vi "report.vi"() -> ()   [LabVIEW 2019, in "database.lvlib"]
uses:
  database.lvlib
  <vilib>/Utility/NIReport.llb/Report Type.ctl
  <vilib>/addons/_office/_exclsub.llb/font.ctl
  <vilib>/Utility/miscctls.llb/LVRowAndColumnTypeDef.ctl
  <vilib>/addons/_office/excel.llb/Excel Easy Table (str).vi
  <vilib>/Utility/NIReport.llb/NI_report.lvclass
  <vilib>/addons/_office/NI_ReportGenerationToolkit.lvlib
  <vilib>/Utility/NIReport.llb/NI_ReportGenerationCore.lvlib
panel:
  in  "Tab Control 1":T1(tab)
  in  "Tab Control 2":T2(tab)
  out "Grading Table Disc 26":string[][](table)
  out "Grading Table Disc 27":string[][](table)
  out "Grading Table Disc 28":string[][](table)
  out "Grading Table Disc 29":string[][](table)
  out "Grading Table Disc 30":string[][](table)
  out "Grading Table Disc 06":string[][](table)
  in  "Search 1":bool
  in  "Print 1":bool
  in  "Close 1":bool
  in  "Save 1":bool
  in  "Tab Control 3":T2(tab)
  out "Main Grading Table Disc 26":string[][](table)
  out "Main Grading Table Disc 27":string[][](table)
  out "Main Grading Table Disc 28":string[][](table)
  out "Main Grading Table Disc 29":string[][](table)
  out "Main Grading Table Disc 30":string[][](table)
  out "Main Grading Table Disc 06":string[][](table)
  in  "Close 2":bool
  in  "Print 2":bool
  in  "Search 2":bool
  in  "Save 2":bool
  out "Log Table":string[][](table)
  out "Log Catalog Table":string[][](table)
  in  "Search 3":bool
  in  "Print 3":bool
  in  "Close 3":bool
  in  "Save 3":bool
  out "User Table":string[][](table)
  in  "Close 4":bool
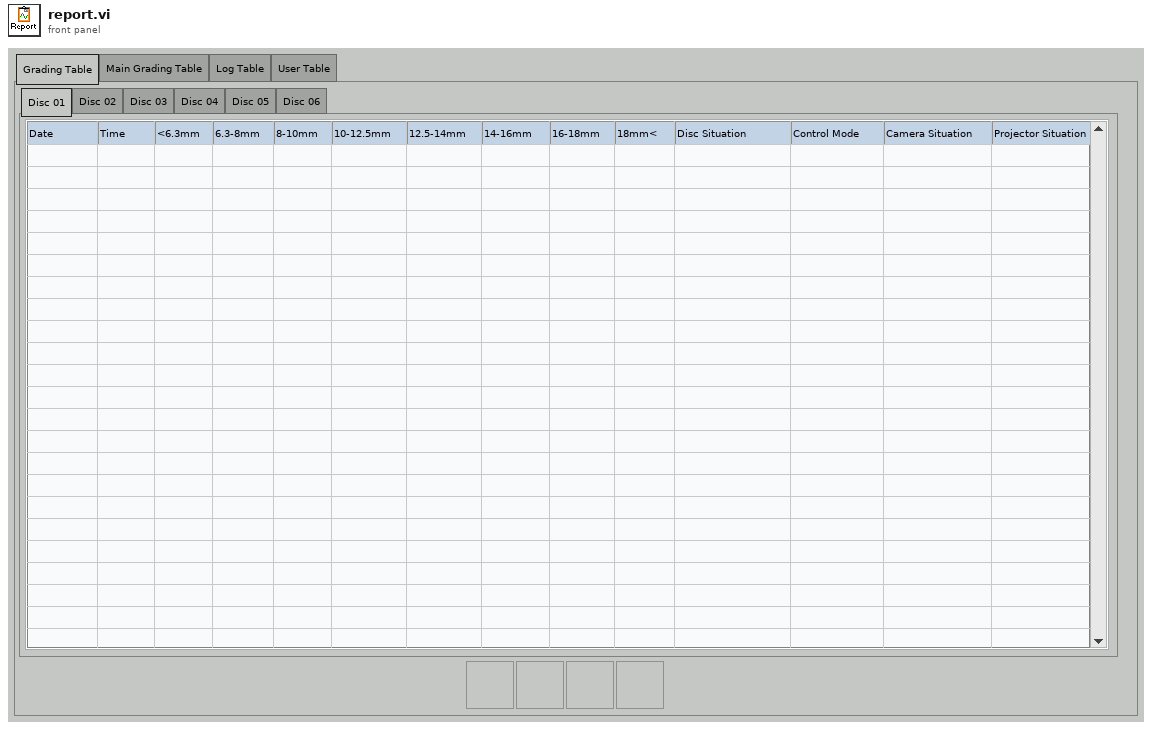
[diagram p1: front panel]
types:
  T1 = enum32{"Grading Table", "Main Grading Table", "Log Table", "User Table"}
  T2 = enum32{"Disc 01", "Disc 02", "Disc 03", "Disc 04", "Disc 05", "Disc 06"}
  T3 = enum16{"None", "On Hover", "On Key Focus", "On Hover or Key Focus"}
  T4 = typedef "NI_ReportGenerationToolkit.lvlib/font.ctl" = cluster{"font name":string, "font size":dbl, "bold":u16, "italic":u16, "underline":u16, "strike through":u16, "font color":u32}
  T5 = typedef "NI_ReportGenerationCore.lvlib/Report Type.ctl" = enum16{"HTML", "Word", "Excel"}
  T6 = enum16{"maximized", "minimized", "normal", "no change"}
  T7 = typedef "LVRowAndColumnTypeDef.ctl" = cluster{"Row":i32, "Column":i32}
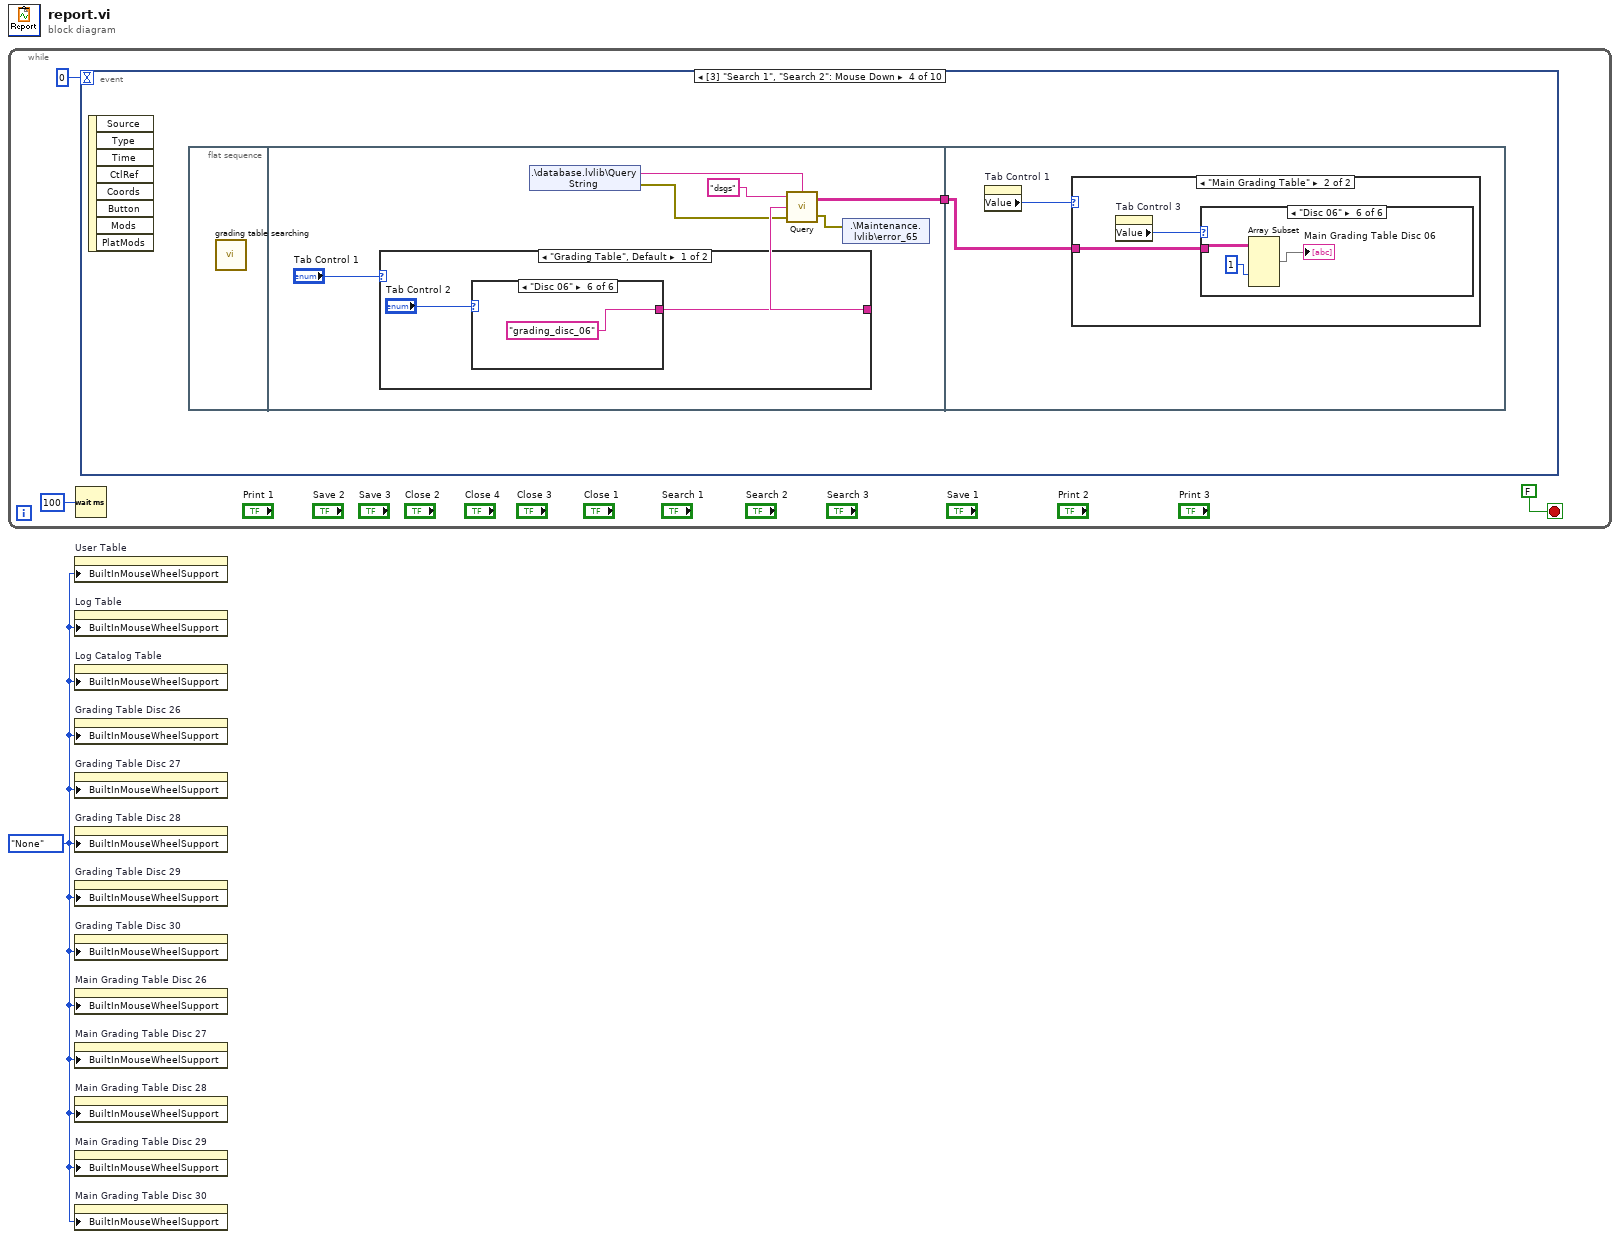
[diagram p0: block diagram]
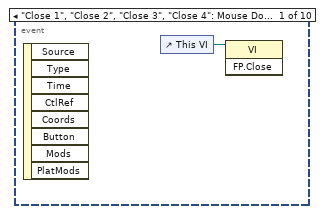
[diagram p2: hidden frame]
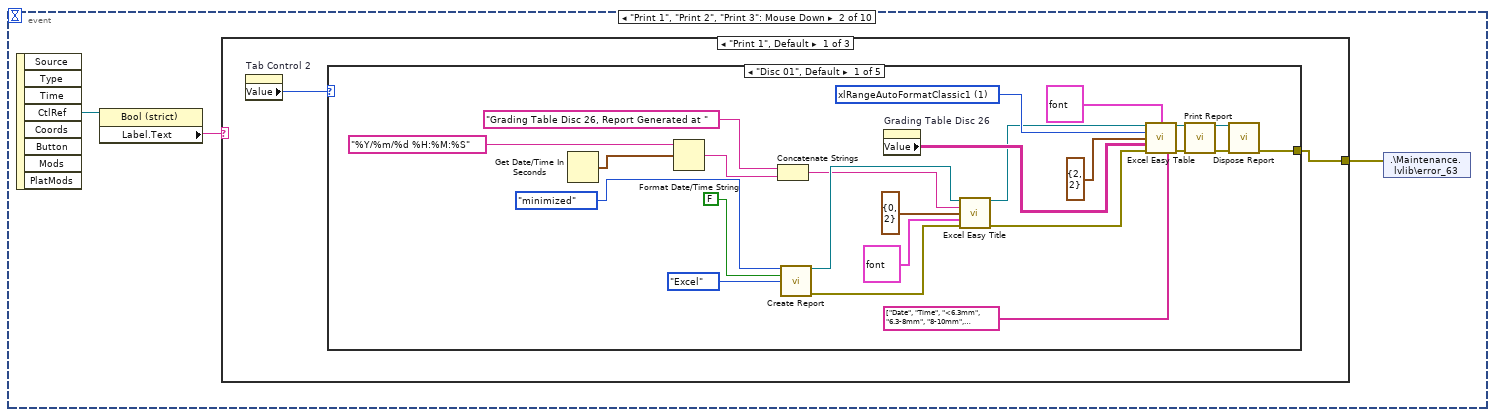
[diagram p3: hidden frame]
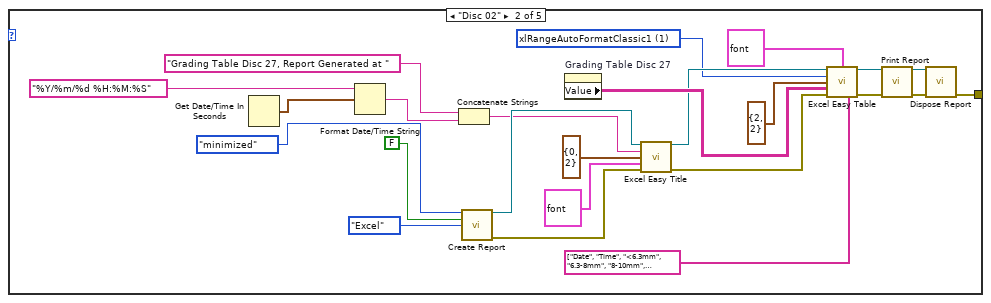
[diagram p4: hidden frame]
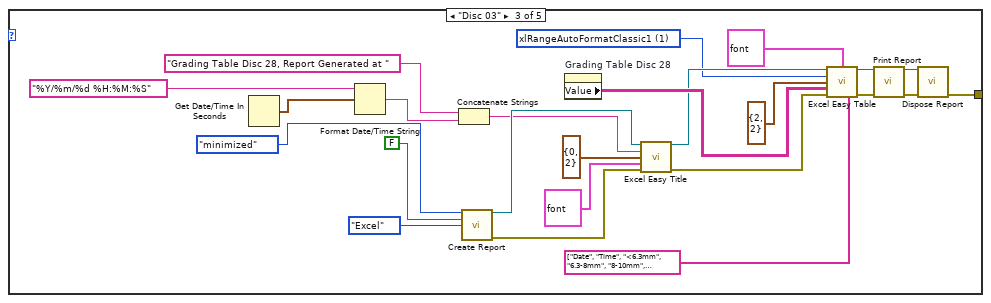
[diagram p5: hidden frame]
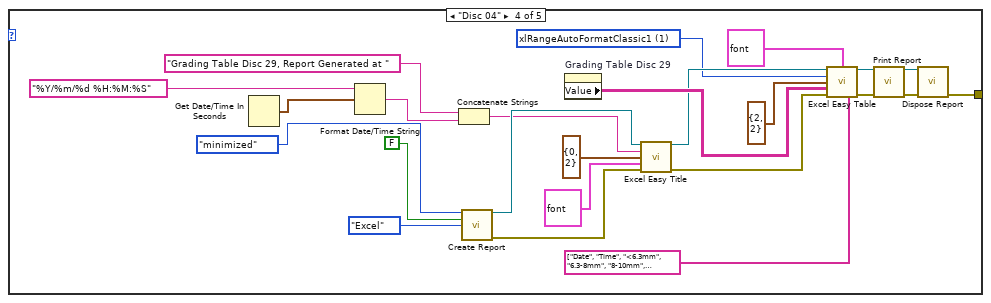
[diagram p6: hidden frame]
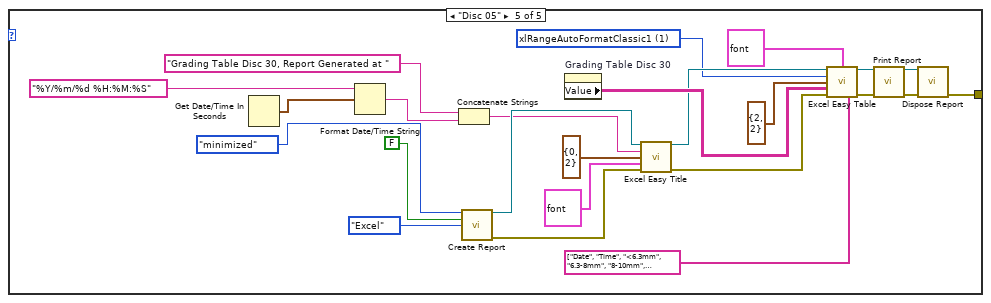
[diagram p7: hidden frame]
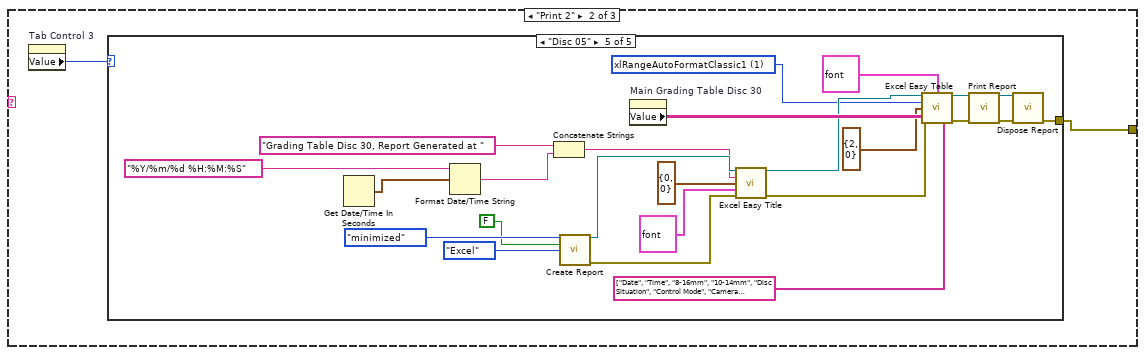
[diagram p8: hidden frame]
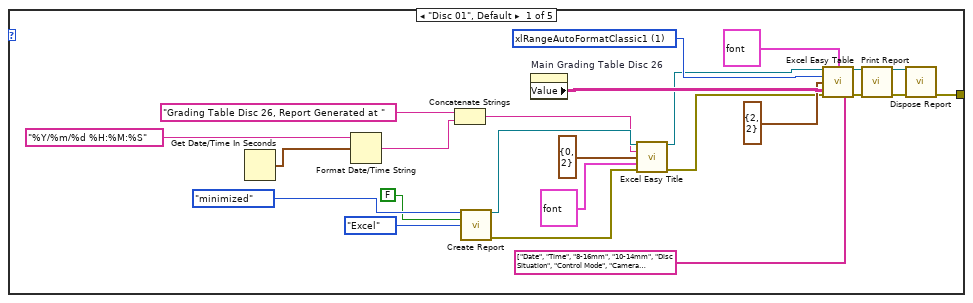
[diagram p9: hidden frame]
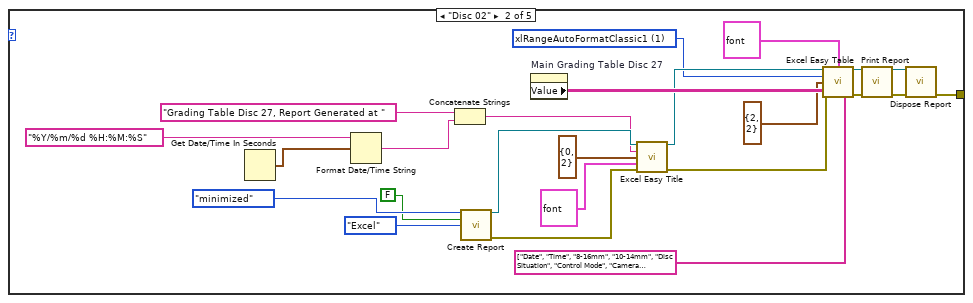
[diagram p10: hidden frame]
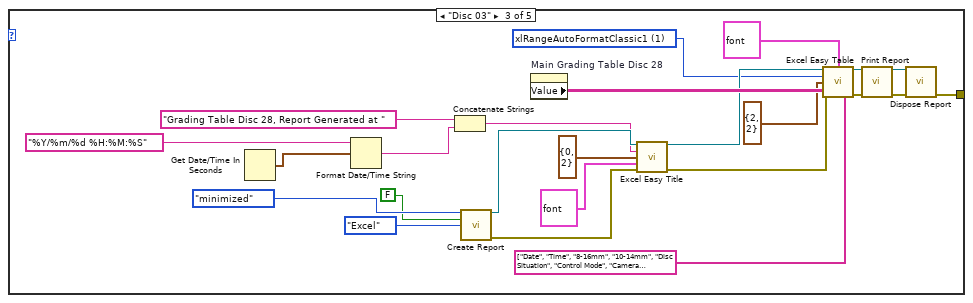
[diagram p11: hidden frame]
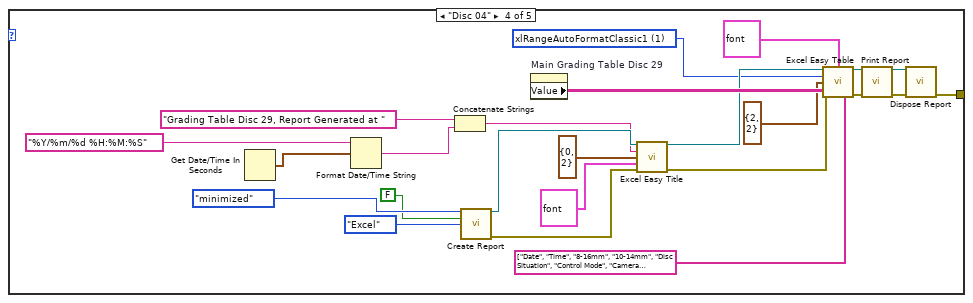
[diagram p12: hidden frame]
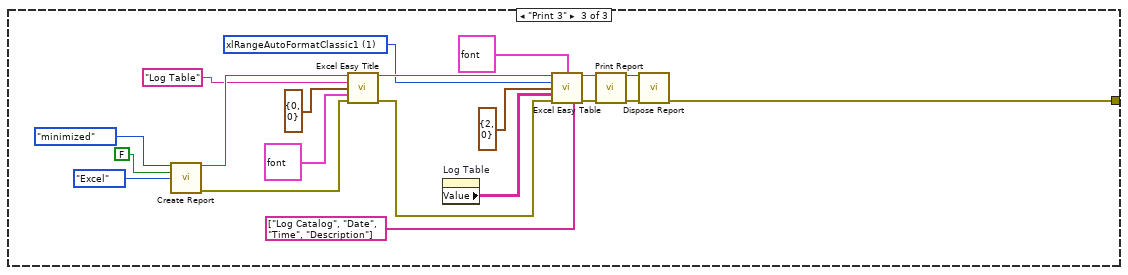
[diagram p13: hidden frame]
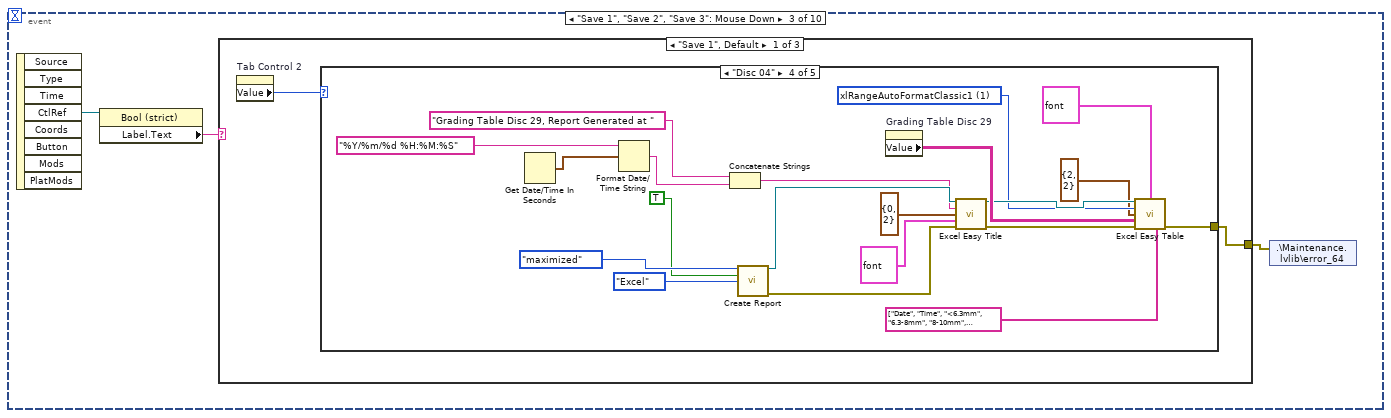
[diagram p14: hidden frame]
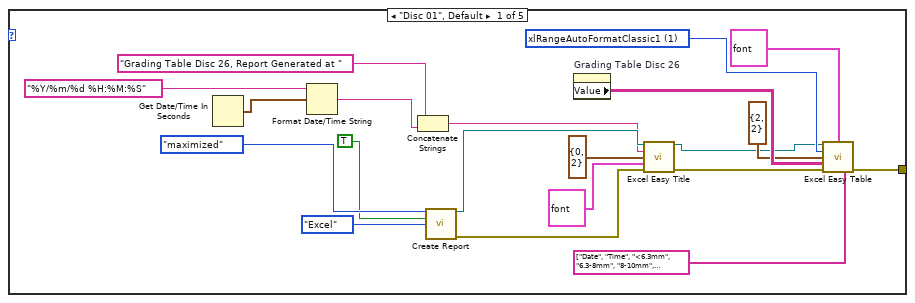
[diagram p15: hidden frame]
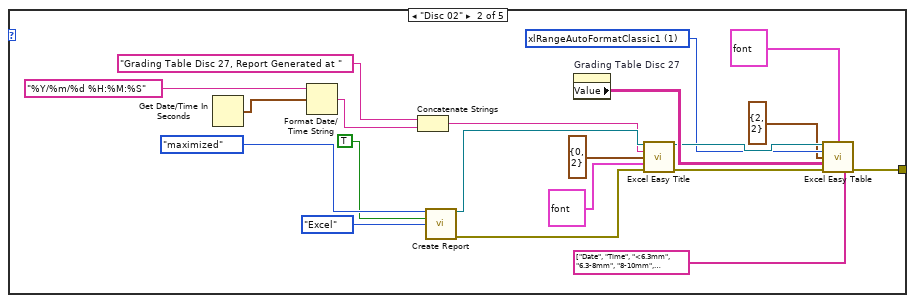
[diagram p16: hidden frame]
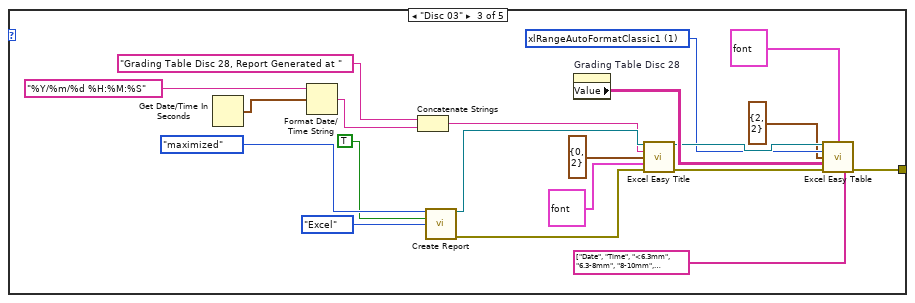
[diagram p17: hidden frame]
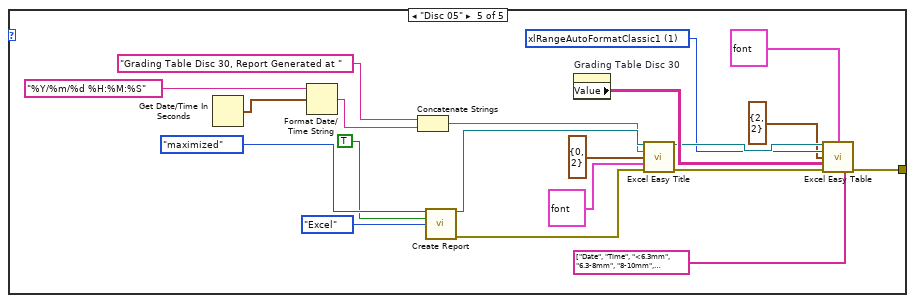
[diagram p18: hidden frame]
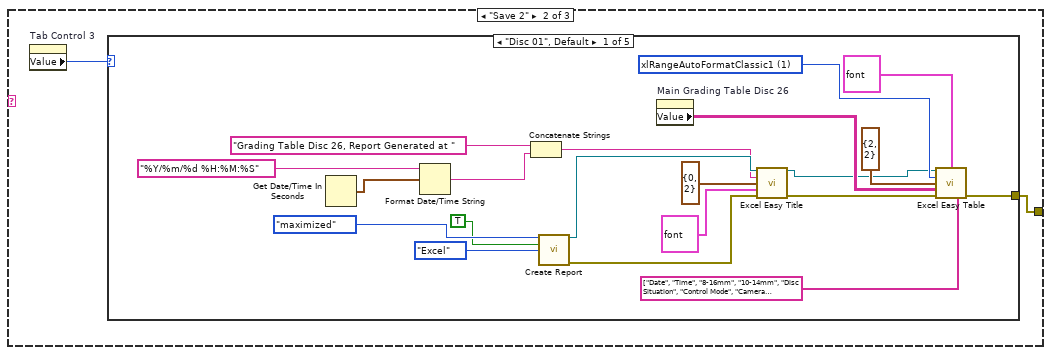
[diagram p19: hidden frame]
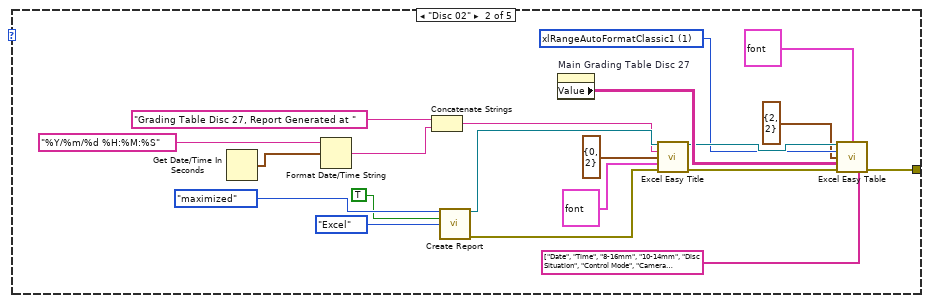
[diagram p20: hidden frame]
diagram:
  w1 = T3."None" ("Built-In Mouse Wheel Support")
  n1 = while {
    stop <- FALSE stop-if-true
    n2 = Wait (ms)(milliseconds to wait=u32 100) -> ()  [unwired: 1 out]
    n3 = event shown="[3] \"Search 1\", \"Search 2\": Mouse Down" {
      selector: _ -> [_ _ _ _ _ _ _ _ _ _]
      dyn-events: _ -> [_ _ _ _ _ _ _ _ _ _]
      timeout: 0 -> [_ _ _ _ _ _ _ _ _ _]
      event "Close 1", "Close 2", "Close 3", "Close 4": Mouse Down {
        n4 = event-data() -> ()  [unwired: 1 in, 8 out]
        n5 = control-ref of="This VI"() -> (w5:refnum<vi>)
        n6 = invoke class="VI" method="FP.Close"(reference=w5) -> ()  [unwired: 2 in, 3 out]
      }
      event "Print 1", "Print 2", "Print 3": Mouse Down {
        n7 = event-data() -> ("CtlRef"=w8:refnum<vi>)  [unwired: 1 in, 7 out]
        n8 = property class="Bool (strict)"(reference=w8) -> ("Label.Text"=w7:string)  [unwired: 1 in, 2 out]
        n9 = case shown="\"Print 1\", Default" w7 {
          tunnel: [w9 w131 w253] -> w6
          frame "Print 1", Default {
            n10 = property on="Tab Control 2" class="TabCtl (strict)"() -> ("Value"=w10:T2)  [unwired: 2 in, 2 out]
            n11 = case shown="\"Disc 01\", Default" w10 {
              tunnel: [w11 w35 w59 w83 w107] -> w9
              frame "Disc 01", Default {
                w28 = 1 items=["xlRangeAutoFormat3DEffects1"=13, "xlRangeAutoFormat3DEffects2"=14, "xlRangeAutoFormatAccounting1"=4, "xlRangeAutoFormatAccounting2"=5, "xlRangeAutoFormatAccounting3"=6, "xlRangeAutoFormatAccounting4"=17, "xlRangeAutoFormatClassic1"=1, "xlRangeAutoFormatClassic2"=2, "xlRangeAutoFormatClassic3"=3, "xlRangeAutoFormatColor1"=7, "xlRangeAutoFormatColor2"=8, "xlRangeAutoFormatColor3"=9, "xlRangeAutoFormatList1"=10, "xlRangeAutoFormatList2"=11, "xlRangeAutoFormatList3"=12, "xlRangeAutoFormatLocalFormat1"=15, "xlRangeAutoFormatLocalFormat2"=16, "xlRangeAutoFormatLocalFormat3"=19, "xlRangeAutoFormatLocalFormat4"=20, "xlRangeAutoFormatReport1"=21, "xlRangeAutoFormatReport2"=22, "xlRangeAutoFormatReport3"=23, "xlRangeAutoFormatReport4"=24, "xlRangeAutoFormatReport5"=25, "xlRangeAutoFormatReport6"=26, "xlRangeAutoFormatReport7"=27, "xlRangeAutoFormatReport8"=28, "xlRangeAutoFormatReport9"=29, "xlRangeAutoFormatReport10"=30, "xlRangeAutoFormatClassicPivotTable"=31, "xlRangeAutoFormatTable1"=32, "xlRangeAutoFormatTable2"=33, "xlRangeAutoFormatTable3"=34, "xlRangeAutoFormatTable4"=35, "xlRangeAutoFormatTable5"=36, "xlRangeAutoFormatTable6"=37, "xlRangeAutoFormatTable7"=38, "xlRangeAutoFormatTable8"=39, "xlRangeAutoFormatTable9"=40, "xlRangeAutoFormatTable10"=41, "xlRangeAutoFormatPTNone"=42, "xlRangeAutoFormatNone"=-4142, "xlRangeAutoFormatSimple"=-4154] ("auto format (none)")
                n12 = Get Date/Time In Seconds() -> (seconds since 1Jan1904=w17:timestamp)
                n13 = Format Date/Time String(time format string (%c)="%Y/%m/%d %H:%M:%S", seconds (now)=w17) -> (date/time string=w18:string)  [unwired: 1 in]
                n14 = Concatenate Strings("Grading Table Disc 26, Report Generated at " ("title"), w18) -> (w19:string)
                n15 = call <vilib>:"Create Report.vi"("window state (normal)"=T6."minimized", "display alerts? (F)"=FALSE, "report type"=Report_Type."Excel") -> ("report out"=w24:refnum<class "NI_report.lvclass">, "error out"=w26:errorcluster)  [unwired: 11 in]
                n16 = property on="Grading Table Disc 26" class="Tbl (strict)"() -> ("Value"=w32:string[][])  [unwired: 2 in, 2 out]
                n17 = call <vilib>:"Excel Easy Title.vi"("report in"=w24, "title"=w19, "start (0, 0)"=cluster{"row":i32, "column":i32} {"row"=0, "column"=2}, "font"=T4 {"font name"="Times New Roman", "font size"=24.0, "bold"=1, "italic"=0, "underline"=0, "strike through"=0, "font color"=16777216}, "error in (no error)"=w26) -> ("report out"=w23:refnum<class "NI_report.lvclass">, "error out"=w25:errorcluster)  [unwired: 8 in, 1 out]
                n18 = call-poly <vilib>:"Excel Easy Table.vi"("report in"=w23, "font"=T4 {"font name"="Times New Roman", "font size"=12.0, "bold"=0, "italic"=0, "underline"=0, "strike through"=0, "font color"=16777216}, "auto format (none)"=w28, "start (0, 0)"=cluster{"row":i32, "column":i32} {"row"=2, "column"=2}, "text data"=w32, "error in (no error)"=w25, "column headers"=string[] ["Date", "Time", "<6.3mm", "6.3-8mm", "8-10mm", "10-12.5mm", "12.5-14mm", "14-16mm", "16-18mm", "18mm<", "Disc Situation", "Control Mode", "Camera Situation", "Projector Situation"]) -> ("report out"=w15:refnum<class "NI_report.lvclass">, "error out"=w14:errorcluster)  [unwired: 4 in, 3 out]
                n19 = call-dynamic "Print Report.vi"("report in"=w15, "error in (no error)"=w14) -> ("report out"=w13:refnum<class "NI_report.lvclass">, "error out"=w12:errorcluster)  [unwired: 12 in]
                n20 = call-dynamic "Dispose Report.vi"("report in"=w13, "error in (no error)"=w12) -> ("error out"=w11:errorcluster)  [unwired: 13 in]
              }
              frame "Disc 02" {
                w42 = 1 items=["xlRangeAutoFormat3DEffects1"=13, "xlRangeAutoFormat3DEffects2"=14, "xlRangeAutoFormatAccounting1"=4, "xlRangeAutoFormatAccounting2"=5, "xlRangeAutoFormatAccounting3"=6, "xlRangeAutoFormatAccounting4"=17, "xlRangeAutoFormatClassic1"=1, "xlRangeAutoFormatClassic2"=2, "xlRangeAutoFormatClassic3"=3, "xlRangeAutoFormatColor1"=7, "xlRangeAutoFormatColor2"=8, "xlRangeAutoFormatColor3"=9, "xlRangeAutoFormatList1"=10, "xlRangeAutoFormatList2"=11, "xlRangeAutoFormatList3"=12, "xlRangeAutoFormatLocalFormat1"=15, "xlRangeAutoFormatLocalFormat2"=16, "xlRangeAutoFormatLocalFormat3"=19, "xlRangeAutoFormatLocalFormat4"=20, "xlRangeAutoFormatReport1"=21, "xlRangeAutoFormatReport2"=22, "xlRangeAutoFormatReport3"=23, "xlRangeAutoFormatReport4"=24, "xlRangeAutoFormatReport5"=25, "xlRangeAutoFormatReport6"=26, "xlRangeAutoFormatReport7"=27, "xlRangeAutoFormatReport8"=28, "xlRangeAutoFormatReport9"=29, "xlRangeAutoFormatReport10"=30, "xlRangeAutoFormatClassicPivotTable"=31, "xlRangeAutoFormatTable1"=32, "xlRangeAutoFormatTable2"=33, "xlRangeAutoFormatTable3"=34, "xlRangeAutoFormatTable4"=35, "xlRangeAutoFormatTable5"=36, "xlRangeAutoFormatTable6"=37, "xlRangeAutoFormatTable7"=38, "xlRangeAutoFormatTable8"=39, "xlRangeAutoFormatTable9"=40, "xlRangeAutoFormatTable10"=41, "xlRangeAutoFormatPTNone"=42, "xlRangeAutoFormatNone"=-4142, "xlRangeAutoFormatSimple"=-4154] ("auto format (none)")
                n21 = Get Date/Time In Seconds() -> (seconds since 1Jan1904=w51:timestamp)
                n22 = Format Date/Time String(time format string (%c)="%Y/%m/%d %H:%M:%S", seconds (now)=w51) -> (date/time string=w52:string)  [unwired: 1 in]
                n23 = Concatenate Strings("Grading Table Disc 27, Report Generated at " ("title"), w52) -> (w53:string)
                n24 = call <vilib>:"Create Report.vi"("window state (normal)"=T6."minimized", "display alerts? (F)"=FALSE, "report type"=Report_Type."Excel") -> ("report out"=w55:refnum<class "NI_report.lvclass">, "error out"=w57:errorcluster)  [unwired: 11 in]
                n25 = property on="Grading Table Disc 27" class="Tbl (strict)"() -> ("Value"=w58:string[][])  [unwired: 2 in, 2 out]
                n26 = call <vilib>:"Excel Easy Title.vi"("report in"=w55, "title"=w53, "start (0, 0)"=cluster{"row":i32, "column":i32} {"row"=0, "column"=2}, "font"=T4 {"font name"="Times New Roman", "font size"=24.0, "bold"=1, "italic"=0, "underline"=0, "strike through"=0, "font color"=16777216}, "error in (no error)"=w57) -> ("report out"=w54:refnum<class "NI_report.lvclass">, "error out"=w56:errorcluster)  [unwired: 8 in, 1 out]
                n27 = call-poly <vilib>:"Excel Easy Table.vi"("report in"=w54, "font"=T4 {"font name"="Times New Roman", "font size"=12.0, "bold"=0, "italic"=0, "underline"=0, "strike through"=0, "font color"=16777216}, "auto format (none)"=w42, "start (0, 0)"=cluster{"row":i32, "column":i32} {"row"=2, "column"=2}, "text data"=w58, "error in (no error)"=w56, "column headers"=string[] ["Date", "Time", "<6.3mm", "6.3-8mm", "8-10mm", "10-12.5mm", "12.5-14mm", "14-16mm", "16-18mm", "18mm<", "Disc Situation", "Control Mode", "Camera Situation", "Projector Situation"]) -> ("report out"=w39:refnum<class "NI_report.lvclass">, "error out"=w38:errorcluster)  [unwired: 4 in, 3 out]
                n28 = call-dynamic "Print Report.vi"("report in"=w39, "error in (no error)"=w38) -> ("report out"=w36:refnum<class "NI_report.lvclass">, "error out"=w37:errorcluster)  [unwired: 12 in]
                n29 = call-dynamic "Dispose Report.vi"("report in"=w36, "error in (no error)"=w37) -> ("error out"=w35:errorcluster)  [unwired: 13 in]
              }
              frame "Disc 03" {
                w66 = 1 items=["xlRangeAutoFormat3DEffects1"=13, "xlRangeAutoFormat3DEffects2"=14, "xlRangeAutoFormatAccounting1"=4, "xlRangeAutoFormatAccounting2"=5, "xlRangeAutoFormatAccounting3"=6, "xlRangeAutoFormatAccounting4"=17, "xlRangeAutoFormatClassic1"=1, "xlRangeAutoFormatClassic2"=2, "xlRangeAutoFormatClassic3"=3, "xlRangeAutoFormatColor1"=7, "xlRangeAutoFormatColor2"=8, "xlRangeAutoFormatColor3"=9, "xlRangeAutoFormatList1"=10, "xlRangeAutoFormatList2"=11, "xlRangeAutoFormatList3"=12, "xlRangeAutoFormatLocalFormat1"=15, "xlRangeAutoFormatLocalFormat2"=16, "xlRangeAutoFormatLocalFormat3"=19, "xlRangeAutoFormatLocalFormat4"=20, "xlRangeAutoFormatReport1"=21, "xlRangeAutoFormatReport2"=22, "xlRangeAutoFormatReport3"=23, "xlRangeAutoFormatReport4"=24, "xlRangeAutoFormatReport5"=25, "xlRangeAutoFormatReport6"=26, "xlRangeAutoFormatReport7"=27, "xlRangeAutoFormatReport8"=28, "xlRangeAutoFormatReport9"=29, "xlRangeAutoFormatReport10"=30, "xlRangeAutoFormatClassicPivotTable"=31, "xlRangeAutoFormatTable1"=32, "xlRangeAutoFormatTable2"=33, "xlRangeAutoFormatTable3"=34, "xlRangeAutoFormatTable4"=35, "xlRangeAutoFormatTable5"=36, "xlRangeAutoFormatTable6"=37, "xlRangeAutoFormatTable7"=38, "xlRangeAutoFormatTable8"=39, "xlRangeAutoFormatTable9"=40, "xlRangeAutoFormatTable10"=41, "xlRangeAutoFormatPTNone"=42, "xlRangeAutoFormatNone"=-4142, "xlRangeAutoFormatSimple"=-4154] ("auto format (none)")
                n30 = Get Date/Time In Seconds() -> (seconds since 1Jan1904=w75:timestamp)
                n31 = Format Date/Time String(time format string (%c)="%Y/%m/%d %H:%M:%S", seconds (now)=w75) -> (date/time string=w76:string)  [unwired: 1 in]
                n32 = Concatenate Strings("Grading Table Disc 28, Report Generated at " ("title"), w76) -> (w77:string)
                n33 = call <vilib>:"Create Report.vi"("window state (normal)"=T6."minimized", "display alerts? (F)"=FALSE, "report type"=Report_Type."Excel") -> ("report out"=w79:refnum<class "NI_report.lvclass">, "error out"=w81:errorcluster)  [unwired: 11 in]
                n34 = property on="Grading Table Disc 28" class="Tbl (strict)"() -> ("Value"=w82:string[][])  [unwired: 2 in, 2 out]
                n35 = call <vilib>:"Excel Easy Title.vi"("report in"=w79, "title"=w77, "start (0, 0)"=cluster{"row":i32, "column":i32} {"row"=0, "column"=2}, "font"=T4 {"font name"="Times New Roman", "font size"=24.0, "bold"=1, "italic"=0, "underline"=0, "strike through"=0, "font color"=16777216}, "error in (no error)"=w81) -> ("report out"=w78:refnum<class "NI_report.lvclass">, "error out"=w80:errorcluster)  [unwired: 8 in, 1 out]
                n36 = call-poly <vilib>:"Excel Easy Table.vi"("report in"=w78, "font"=T4 {"font name"="Times New Roman", "font size"=12.0, "bold"=0, "italic"=0, "underline"=0, "strike through"=0, "font color"=16777216}, "auto format (none)"=w66, "start (0, 0)"=cluster{"row":i32, "column":i32} {"row"=2, "column"=2}, "text data"=w82, "error in (no error)"=w80, "column headers"=string[] ["Date", "Time", "<6.3mm", "6.3-8mm", "8-10mm", "10-12.5mm", "12.5-14mm", "14-16mm", "16-18mm", "18mm<", "Disc Situation", "Control Mode", "Camera Situation", "Projector Situation"]) -> ("report out"=w63:refnum<class "NI_report.lvclass">, "error out"=w62:errorcluster)  [unwired: 4 in, 3 out]
                n37 = call-dynamic "Print Report.vi"("report in"=w63, "error in (no error)"=w62) -> ("report out"=w60:refnum<class "NI_report.lvclass">, "error out"=w61:errorcluster)  [unwired: 12 in]
                n38 = call-dynamic "Dispose Report.vi"("report in"=w60, "error in (no error)"=w61) -> ("error out"=w59:errorcluster)  [unwired: 13 in]
              }
              frame "Disc 04" {
                w90 = 1 items=["xlRangeAutoFormat3DEffects1"=13, "xlRangeAutoFormat3DEffects2"=14, "xlRangeAutoFormatAccounting1"=4, "xlRangeAutoFormatAccounting2"=5, "xlRangeAutoFormatAccounting3"=6, "xlRangeAutoFormatAccounting4"=17, "xlRangeAutoFormatClassic1"=1, "xlRangeAutoFormatClassic2"=2, "xlRangeAutoFormatClassic3"=3, "xlRangeAutoFormatColor1"=7, "xlRangeAutoFormatColor2"=8, "xlRangeAutoFormatColor3"=9, "xlRangeAutoFormatList1"=10, "xlRangeAutoFormatList2"=11, "xlRangeAutoFormatList3"=12, "xlRangeAutoFormatLocalFormat1"=15, "xlRangeAutoFormatLocalFormat2"=16, "xlRangeAutoFormatLocalFormat3"=19, "xlRangeAutoFormatLocalFormat4"=20, "xlRangeAutoFormatReport1"=21, "xlRangeAutoFormatReport2"=22, "xlRangeAutoFormatReport3"=23, "xlRangeAutoFormatReport4"=24, "xlRangeAutoFormatReport5"=25, "xlRangeAutoFormatReport6"=26, "xlRangeAutoFormatReport7"=27, "xlRangeAutoFormatReport8"=28, "xlRangeAutoFormatReport9"=29, "xlRangeAutoFormatReport10"=30, "xlRangeAutoFormatClassicPivotTable"=31, "xlRangeAutoFormatTable1"=32, "xlRangeAutoFormatTable2"=33, "xlRangeAutoFormatTable3"=34, "xlRangeAutoFormatTable4"=35, "xlRangeAutoFormatTable5"=36, "xlRangeAutoFormatTable6"=37, "xlRangeAutoFormatTable7"=38, "xlRangeAutoFormatTable8"=39, "xlRangeAutoFormatTable9"=40, "xlRangeAutoFormatTable10"=41, "xlRangeAutoFormatPTNone"=42, "xlRangeAutoFormatNone"=-4142, "xlRangeAutoFormatSimple"=-4154] ("auto format (none)")
                n39 = Get Date/Time In Seconds() -> (seconds since 1Jan1904=w99:timestamp)
                n40 = Format Date/Time String(time format string (%c)="%Y/%m/%d %H:%M:%S", seconds (now)=w99) -> (date/time string=w100:string)  [unwired: 1 in]
                n41 = Concatenate Strings("Grading Table Disc 29, Report Generated at " ("title"), w100) -> (w101:string)
                n42 = call <vilib>:"Create Report.vi"("window state (normal)"=T6."minimized", "display alerts? (F)"=FALSE, "report type"=Report_Type."Excel") -> ("report out"=w103:refnum<class "NI_report.lvclass">, "error out"=w105:errorcluster)  [unwired: 11 in]
                n43 = property on="Grading Table Disc 29" class="Tbl (strict)"() -> ("Value"=w106:string[][])  [unwired: 2 in, 2 out]
                n44 = call <vilib>:"Excel Easy Title.vi"("report in"=w103, "title"=w101, "start (0, 0)"=cluster{"row":i32, "column":i32} {"row"=0, "column"=2}, "font"=T4 {"font name"="Times New Roman", "font size"=24.0, "bold"=1, "italic"=0, "underline"=0, "strike through"=0, "font color"=16777216}, "error in (no error)"=w105) -> ("report out"=w102:refnum<class "NI_report.lvclass">, "error out"=w104:errorcluster)  [unwired: 8 in, 1 out]
                n45 = call-poly <vilib>:"Excel Easy Table.vi"("report in"=w102, "font"=T4 {"font name"="Times New Roman", "font size"=12.0, "bold"=0, "italic"=0, "underline"=0, "strike through"=0, "font color"=16777216}, "auto format (none)"=w90, "start (0, 0)"=cluster{"row":i32, "column":i32} {"row"=2, "column"=2}, "text data"=w106, "error in (no error)"=w104, "column headers"=string[] ["Date", "Time", "<6.3mm", "6.3-8mm", "8-10mm", "10-12.5mm", "12.5-14mm", "14-16mm", "16-18mm", "18mm<", "Disc Situation", "Control Mode", "Camera Situation", "Projector Situation"]) -> ("report out"=w87:refnum<class "NI_report.lvclass">, "error out"=w86:errorcluster)  [unwired: 4 in, 3 out]
                n46 = call-dynamic "Print Report.vi"("report in"=w87, "error in (no error)"=w86) -> ("report out"=w84:refnum<class "NI_report.lvclass">, "error out"=w85:errorcluster)  [unwired: 12 in]
                n47 = call-dynamic "Dispose Report.vi"("report in"=w84, "error in (no error)"=w85) -> ("error out"=w83:errorcluster)  [unwired: 13 in]
              }
              frame "Disc 05" {
                w114 = 1 items=["xlRangeAutoFormat3DEffects1"=13, "xlRangeAutoFormat3DEffects2"=14, "xlRangeAutoFormatAccounting1"=4, "xlRangeAutoFormatAccounting2"=5, "xlRangeAutoFormatAccounting3"=6, "xlRangeAutoFormatAccounting4"=17, "xlRangeAutoFormatClassic1"=1, "xlRangeAutoFormatClassic2"=2, "xlRangeAutoFormatClassic3"=3, "xlRangeAutoFormatColor1"=7, "xlRangeAutoFormatColor2"=8, "xlRangeAutoFormatColor3"=9, "xlRangeAutoFormatList1"=10, "xlRangeAutoFormatList2"=11, "xlRangeAutoFormatList3"=12, "xlRangeAutoFormatLocalFormat1"=15, "xlRangeAutoFormatLocalFormat2"=16, "xlRangeAutoFormatLocalFormat3"=19, "xlRangeAutoFormatLocalFormat4"=20, "xlRangeAutoFormatReport1"=21, "xlRangeAutoFormatReport2"=22, "xlRangeAutoFormatReport3"=23, "xlRangeAutoFormatReport4"=24, "xlRangeAutoFormatReport5"=25, "xlRangeAutoFormatReport6"=26, "xlRangeAutoFormatReport7"=27, "xlRangeAutoFormatReport8"=28, "xlRangeAutoFormatReport9"=29, "xlRangeAutoFormatReport10"=30, "xlRangeAutoFormatClassicPivotTable"=31, "xlRangeAutoFormatTable1"=32, "xlRangeAutoFormatTable2"=33, "xlRangeAutoFormatTable3"=34, "xlRangeAutoFormatTable4"=35, "xlRangeAutoFormatTable5"=36, "xlRangeAutoFormatTable6"=37, "xlRangeAutoFormatTable7"=38, "xlRangeAutoFormatTable8"=39, "xlRangeAutoFormatTable9"=40, "xlRangeAutoFormatTable10"=41, "xlRangeAutoFormatPTNone"=42, "xlRangeAutoFormatNone"=-4142, "xlRangeAutoFormatSimple"=-4154] ("auto format (none)")
                n48 = Get Date/Time In Seconds() -> (seconds since 1Jan1904=w123:timestamp)
                n49 = Format Date/Time String(time format string (%c)="%Y/%m/%d %H:%M:%S", seconds (now)=w123) -> (date/time string=w124:string)  [unwired: 1 in]
                n50 = Concatenate Strings("Grading Table Disc 30, Report Generated at " ("title"), w124) -> (w125:string)
                n51 = call <vilib>:"Create Report.vi"("window state (normal)"=T6."minimized", "display alerts? (F)"=FALSE, "report type"=Report_Type."Excel") -> ("report out"=w127:refnum<class "NI_report.lvclass">, "error out"=w129:errorcluster)  [unwired: 11 in]
                n52 = property on="Grading Table Disc 30" class="Tbl (strict)"() -> ("Value"=w130:string[][])  [unwired: 2 in, 2 out]
                n53 = call <vilib>:"Excel Easy Title.vi"("report in"=w127, "title"=w125, "start (0, 0)"=cluster{"row":i32, "column":i32} {"row"=0, "column"=2}, "font"=T4 {"font name"="Times New Roman", "font size"=24.0, "bold"=1, "italic"=0, "underline"=0, "strike through"=0, "font color"=16777216}, "error in (no error)"=w129) -> ("report out"=w126:refnum<class "NI_report.lvclass">, "error out"=w128:errorcluster)  [unwired: 8 in, 1 out]
                n54 = call-poly <vilib>:"Excel Easy Table.vi"("report in"=w126, "font"=T4 {"font name"="Times New Roman", "font size"=12.0, "bold"=0, "italic"=0, "underline"=0, "strike through"=0, "font color"=16777216}, "auto format (none)"=w114, "start (0, 0)"=cluster{"row":i32, "column":i32} {"row"=2, "column"=2}, "text data"=w130, "error in (no error)"=w128, "column headers"=string[] ["Date", "Time", "<6.3mm", "6.3-8mm", "8-10mm", "10-12.5mm", "12.5-14mm", "14-16mm", "16-18mm", "18mm<", "Disc Situation", "Control Mode", "Camera Situation", "Projector Situation"]) -> ("report out"=w110:refnum<class "NI_report.lvclass">, "error out"=w111:errorcluster)  [unwired: 4 in, 3 out]
                n55 = call-dynamic "Print Report.vi"("report in"=w110, "error in (no error)"=w111) -> ("report out"=w108:refnum<class "NI_report.lvclass">, "error out"=w109:errorcluster)  [unwired: 12 in]
                n56 = call-dynamic "Dispose Report.vi"("report in"=w108, "error in (no error)"=w109) -> ("error out"=w107:errorcluster)  [unwired: 13 in]
              }
            }
          }
          frame "Print 2" {
            n57 = property on="Tab Control 3" class="TabCtl (strict)"() -> ("Value"=w132:T2)  [unwired: 2 in, 2 out]
            n58 = case shown="\"Disc 05\"" w132 {
              tunnel: [w133 w157 w181 w205 w229] -> w131
              frame "Disc 01", Default {
                w151 = 1 items=["xlRangeAutoFormat3DEffects1"=13, "xlRangeAutoFormat3DEffects2"=14, "xlRangeAutoFormatAccounting1"=4, "xlRangeAutoFormatAccounting2"=5, "xlRangeAutoFormatAccounting3"=6, "xlRangeAutoFormatAccounting4"=17, "xlRangeAutoFormatClassic1"=1, "xlRangeAutoFormatClassic2"=2, "xlRangeAutoFormatClassic3"=3, "xlRangeAutoFormatColor1"=7, "xlRangeAutoFormatColor2"=8, "xlRangeAutoFormatColor3"=9, "xlRangeAutoFormatList1"=10, "xlRangeAutoFormatList2"=11, "xlRangeAutoFormatList3"=12, "xlRangeAutoFormatLocalFormat1"=15, "xlRangeAutoFormatLocalFormat2"=16, "xlRangeAutoFormatLocalFormat3"=19, "xlRangeAutoFormatLocalFormat4"=20, "xlRangeAutoFormatReport1"=21, "xlRangeAutoFormatReport2"=22, "xlRangeAutoFormatReport3"=23, "xlRangeAutoFormatReport4"=24, "xlRangeAutoFormatReport5"=25, "xlRangeAutoFormatReport6"=26, "xlRangeAutoFormatReport7"=27, "xlRangeAutoFormatReport8"=28, "xlRangeAutoFormatReport9"=29, "xlRangeAutoFormatReport10"=30, "xlRangeAutoFormatClassicPivotTable"=31, "xlRangeAutoFormatTable1"=32, "xlRangeAutoFormatTable2"=33, "xlRangeAutoFormatTable3"=34, "xlRangeAutoFormatTable4"=35, "xlRangeAutoFormatTable5"=36, "xlRangeAutoFormatTable6"=37, "xlRangeAutoFormatTable7"=38, "xlRangeAutoFormatTable8"=39, "xlRangeAutoFormatTable9"=40, "xlRangeAutoFormatTable10"=41, "xlRangeAutoFormatPTNone"=42, "xlRangeAutoFormatNone"=-4142, "xlRangeAutoFormatSimple"=-4154] ("auto format (none)")
                n59 = Get Date/Time In Seconds() -> (seconds since 1Jan1904=w140:timestamp)
                n60 = Format Date/Time String(time format string (%c)="%Y/%m/%d %H:%M:%S", seconds (now)=w140) -> (date/time string=w141:string)  [unwired: 1 in]
                n61 = Concatenate Strings("Grading Table Disc 26, Report Generated at " ("title"), w141) -> (w142:string)
                n62 = call <vilib>:"Create Report.vi"("window state (normal)"=T6."minimized", "display alerts? (F)"=FALSE, "report type"=Report_Type."Excel") -> ("report out"=w147:refnum<class "NI_report.lvclass">, "error out"=w149:errorcluster)  [unwired: 11 in]
                n63 = property on="Main Grading Table Disc 26" class="Tbl (strict)"() -> ("Value"=w154:string[][])  [unwired: 2 in, 2 out]
                n64 = call <vilib>:"Excel Easy Title.vi"("report in"=w147, "title"=w142, "start (0, 0)"=cluster{"row":i32, "column":i32} {"row"=0, "column"=2}, "font"=T4 {"font name"="Times New Roman", "font size"=24.0, "bold"=1, "italic"=0, "underline"=0, "strike through"=0, "font color"=16777216}, "error in (no error)"=w149) -> ("report out"=w146:refnum<class "NI_report.lvclass">, "error out"=w148:errorcluster)  [unwired: 8 in, 1 out]
                n65 = call-poly <vilib>:"Excel Easy Table.vi"("report in"=w146, "font"=T4 {"font name"="Times New Roman", "font size"=12.0, "bold"=0, "italic"=0, "underline"=0, "strike through"=0, "font color"=16777216}, "auto format (none)"=w151, "start (0, 0)"=cluster{"row":i32, "column":i32} {"row"=2, "column"=2}, "text data"=w154, "error in (no error)"=w148, "column headers"=string[] ["Date", "Time", "8-16mm", "10-14mm", "Disc Situation", "Control Mode", "Camera Situation", "Projector Situation"]) -> ("report out"=w136:refnum<class "NI_report.lvclass">, "error out"=w137:errorcluster)  [unwired: 4 in, 3 out]
                n66 = call-dynamic "Print Report.vi"("report in"=w136, "error in (no error)"=w137) -> ("report out"=w134:refnum<class "NI_report.lvclass">, "error out"=w135:errorcluster)  [unwired: 12 in]
                n67 = call-dynamic "Dispose Report.vi"("report in"=w134, "error in (no error)"=w135) -> ("error out"=w133:errorcluster)  [unwired: 13 in]
              }
              frame "Disc 02" {
                w164 = 1 items=["xlRangeAutoFormat3DEffects1"=13, "xlRangeAutoFormat3DEffects2"=14, "xlRangeAutoFormatAccounting1"=4, "xlRangeAutoFormatAccounting2"=5, "xlRangeAutoFormatAccounting3"=6, "xlRangeAutoFormatAccounting4"=17, "xlRangeAutoFormatClassic1"=1, "xlRangeAutoFormatClassic2"=2, "xlRangeAutoFormatClassic3"=3, "xlRangeAutoFormatColor1"=7, "xlRangeAutoFormatColor2"=8, "xlRangeAutoFormatColor3"=9, "xlRangeAutoFormatList1"=10, "xlRangeAutoFormatList2"=11, "xlRangeAutoFormatList3"=12, "xlRangeAutoFormatLocalFormat1"=15, "xlRangeAutoFormatLocalFormat2"=16, "xlRangeAutoFormatLocalFormat3"=19, "xlRangeAutoFormatLocalFormat4"=20, "xlRangeAutoFormatReport1"=21, "xlRangeAutoFormatReport2"=22, "xlRangeAutoFormatReport3"=23, "xlRangeAutoFormatReport4"=24, "xlRangeAutoFormatReport5"=25, "xlRangeAutoFormatReport6"=26, "xlRangeAutoFormatReport7"=27, "xlRangeAutoFormatReport8"=28, "xlRangeAutoFormatReport9"=29, "xlRangeAutoFormatReport10"=30, "xlRangeAutoFormatClassicPivotTable"=31, "xlRangeAutoFormatTable1"=32, "xlRangeAutoFormatTable2"=33, "xlRangeAutoFormatTable3"=34, "xlRangeAutoFormatTable4"=35, "xlRangeAutoFormatTable5"=36, "xlRangeAutoFormatTable6"=37, "xlRangeAutoFormatTable7"=38, "xlRangeAutoFormatTable8"=39, "xlRangeAutoFormatTable9"=40, "xlRangeAutoFormatTable10"=41, "xlRangeAutoFormatPTNone"=42, "xlRangeAutoFormatNone"=-4142, "xlRangeAutoFormatSimple"=-4154] ("auto format (none)")
                n68 = Get Date/Time In Seconds() -> (seconds since 1Jan1904=w173:timestamp)
                n69 = Format Date/Time String(time format string (%c)="%Y/%m/%d %H:%M:%S", seconds (now)=w173) -> (date/time string=w174:string)  [unwired: 1 in]
                n70 = Concatenate Strings("Grading Table Disc 27, Report Generated at " ("title"), w174) -> (w175:string)
                n71 = call <vilib>:"Create Report.vi"("window state (normal)"=T6."minimized", "display alerts? (F)"=FALSE, "report type"=Report_Type."Excel") -> ("report out"=w177:refnum<class "NI_report.lvclass">, "error out"=w179:errorcluster)  [unwired: 11 in]
                n72 = property on="Main Grading Table Disc 27" class="Tbl (strict)"() -> ("Value"=w180:string[][])  [unwired: 2 in, 2 out]
                n73 = call <vilib>:"Excel Easy Title.vi"("report in"=w177, "title"=w175, "start (0, 0)"=cluster{"row":i32, "column":i32} {"row"=0, "column"=2}, "font"=T4 {"font name"="Times New Roman", "font size"=24.0, "bold"=1, "italic"=0, "underline"=0, "strike through"=0, "font color"=16777216}, "error in (no error)"=w179) -> ("report out"=w176:refnum<class "NI_report.lvclass">, "error out"=w178:errorcluster)  [unwired: 8 in, 1 out]
                n74 = call-poly <vilib>:"Excel Easy Table.vi"("report in"=w176, "font"=T4 {"font name"="Times New Roman", "font size"=12.0, "bold"=0, "italic"=0, "underline"=0, "strike through"=0, "font color"=16777216}, "auto format (none)"=w164, "start (0, 0)"=cluster{"row":i32, "column":i32} {"row"=2, "column"=2}, "text data"=w180, "error in (no error)"=w178, "column headers"=string[] ["Date", "Time", "8-16mm", "10-14mm", "Disc Situation", "Control Mode", "Camera Situation", "Projector Situation"]) -> ("report out"=w160:refnum<class "NI_report.lvclass">, "error out"=w161:errorcluster)  [unwired: 4 in, 3 out]
                n75 = call-dynamic "Print Report.vi"("report in"=w160, "error in (no error)"=w161) -> ("report out"=w158:refnum<class "NI_report.lvclass">, "error out"=w159:errorcluster)  [unwired: 12 in]
                n76 = call-dynamic "Dispose Report.vi"("report in"=w158, "error in (no error)"=w159) -> ("error out"=w157:errorcluster)  [unwired: 13 in]
              }
              frame "Disc 03" {
                w188 = 1 items=["xlRangeAutoFormat3DEffects1"=13, "xlRangeAutoFormat3DEffects2"=14, "xlRangeAutoFormatAccounting1"=4, "xlRangeAutoFormatAccounting2"=5, "xlRangeAutoFormatAccounting3"=6, "xlRangeAutoFormatAccounting4"=17, "xlRangeAutoFormatClassic1"=1, "xlRangeAutoFormatClassic2"=2, "xlRangeAutoFormatClassic3"=3, "xlRangeAutoFormatColor1"=7, "xlRangeAutoFormatColor2"=8, "xlRangeAutoFormatColor3"=9, "xlRangeAutoFormatList1"=10, "xlRangeAutoFormatList2"=11, "xlRangeAutoFormatList3"=12, "xlRangeAutoFormatLocalFormat1"=15, "xlRangeAutoFormatLocalFormat2"=16, "xlRangeAutoFormatLocalFormat3"=19, "xlRangeAutoFormatLocalFormat4"=20, "xlRangeAutoFormatReport1"=21, "xlRangeAutoFormatReport2"=22, "xlRangeAutoFormatReport3"=23, "xlRangeAutoFormatReport4"=24, "xlRangeAutoFormatReport5"=25, "xlRangeAutoFormatReport6"=26, "xlRangeAutoFormatReport7"=27, "xlRangeAutoFormatReport8"=28, "xlRangeAutoFormatReport9"=29, "xlRangeAutoFormatReport10"=30, "xlRangeAutoFormatClassicPivotTable"=31, "xlRangeAutoFormatTable1"=32, "xlRangeAutoFormatTable2"=33, "xlRangeAutoFormatTable3"=34, "xlRangeAutoFormatTable4"=35, "xlRangeAutoFormatTable5"=36, "xlRangeAutoFormatTable6"=37, "xlRangeAutoFormatTable7"=38, "xlRangeAutoFormatTable8"=39, "xlRangeAutoFormatTable9"=40, "xlRangeAutoFormatTable10"=41, "xlRangeAutoFormatPTNone"=42, "xlRangeAutoFormatNone"=-4142, "xlRangeAutoFormatSimple"=-4154] ("auto format (none)")
                n77 = Get Date/Time In Seconds() -> (seconds since 1Jan1904=w197:timestamp)
                n78 = Format Date/Time String(time format string (%c)="%Y/%m/%d %H:%M:%S", seconds (now)=w197) -> (date/time string=w198:string)  [unwired: 1 in]
                n79 = Concatenate Strings("Grading Table Disc 28, Report Generated at " ("title"), w198) -> (w199:string)
                n80 = call <vilib>:"Create Report.vi"("window state (normal)"=T6."minimized", "display alerts? (F)"=FALSE, "report type"=Report_Type."Excel") -> ("report out"=w201:refnum<class "NI_report.lvclass">, "error out"=w203:errorcluster)  [unwired: 11 in]
                n81 = property on="Main Grading Table Disc 28" class="Tbl (strict)"() -> ("Value"=w204:string[][])  [unwired: 2 in, 2 out]
                n82 = call <vilib>:"Excel Easy Title.vi"("report in"=w201, "title"=w199, "start (0, 0)"=cluster{"row":i32, "column":i32} {"row"=0, "column"=2}, "font"=T4 {"font name"="Times New Roman", "font size"=24.0, "bold"=1, "italic"=0, "underline"=0, "strike through"=0, "font color"=16777216}, "error in (no error)"=w203) -> ("report out"=w200:refnum<class "NI_report.lvclass">, "error out"=w202:errorcluster)  [unwired: 8 in, 1 out]
                n83 = call-poly <vilib>:"Excel Easy Table.vi"("report in"=w200, "font"=T4 {"font name"="Times New Roman", "font size"=12.0, "bold"=0, "italic"=0, "underline"=0, "strike through"=0, "font color"=16777216}, "auto format (none)"=w188, "start (0, 0)"=cluster{"row":i32, "column":i32} {"row"=2, "column"=2}, "text data"=w204, "error in (no error)"=w202, "column headers"=string[] ["Date", "Time", "8-16mm", "10-14mm", "Disc Situation", "Control Mode", "Camera Situation", "Projector Situation"]) -> ("report out"=w184:refnum<class "NI_report.lvclass">, "error out"=w185:errorcluster)  [unwired: 4 in, 3 out]
                n84 = call-dynamic "Print Report.vi"("report in"=w184, "error in (no error)"=w185) -> ("report out"=w182:refnum<class "NI_report.lvclass">, "error out"=w183:errorcluster)  [unwired: 12 in]
                n85 = call-dynamic "Dispose Report.vi"("report in"=w182, "error in (no error)"=w183) -> ("error out"=w181:errorcluster)  [unwired: 13 in]
              }
              frame "Disc 04" {
                w212 = 1 items=["xlRangeAutoFormat3DEffects1"=13, "xlRangeAutoFormat3DEffects2"=14, "xlRangeAutoFormatAccounting1"=4, "xlRangeAutoFormatAccounting2"=5, "xlRangeAutoFormatAccounting3"=6, "xlRangeAutoFormatAccounting4"=17, "xlRangeAutoFormatClassic1"=1, "xlRangeAutoFormatClassic2"=2, "xlRangeAutoFormatClassic3"=3, "xlRangeAutoFormatColor1"=7, "xlRangeAutoFormatColor2"=8, "xlRangeAutoFormatColor3"=9, "xlRangeAutoFormatList1"=10, "xlRangeAutoFormatList2"=11, "xlRangeAutoFormatList3"=12, "xlRangeAutoFormatLocalFormat1"=15, "xlRangeAutoFormatLocalFormat2"=16, "xlRangeAutoFormatLocalFormat3"=19, "xlRangeAutoFormatLocalFormat4"=20, "xlRangeAutoFormatReport1"=21, "xlRangeAutoFormatReport2"=22, "xlRangeAutoFormatReport3"=23, "xlRangeAutoFormatReport4"=24, "xlRangeAutoFormatReport5"=25, "xlRangeAutoFormatReport6"=26, "xlRangeAutoFormatReport7"=27, "xlRangeAutoFormatReport8"=28, "xlRangeAutoFormatReport9"=29, "xlRangeAutoFormatReport10"=30, "xlRangeAutoFormatClassicPivotTable"=31, "xlRangeAutoFormatTable1"=32, "xlRangeAutoFormatTable2"=33, "xlRangeAutoFormatTable3"=34, "xlRangeAutoFormatTable4"=35, "xlRangeAutoFormatTable5"=36, "xlRangeAutoFormatTable6"=37, "xlRangeAutoFormatTable7"=38, "xlRangeAutoFormatTable8"=39, "xlRangeAutoFormatTable9"=40, "xlRangeAutoFormatTable10"=41, "xlRangeAutoFormatPTNone"=42, "xlRangeAutoFormatNone"=-4142, "xlRangeAutoFormatSimple"=-4154] ("auto format (none)")
                n86 = Get Date/Time In Seconds() -> (seconds since 1Jan1904=w221:timestamp)
                n87 = Format Date/Time String(time format string (%c)="%Y/%m/%d %H:%M:%S", seconds (now)=w221) -> (date/time string=w222:string)  [unwired: 1 in]
                n88 = Concatenate Strings("Grading Table Disc 29, Report Generated at " ("title"), w222) -> (w223:string)
                n89 = call <vilib>:"Create Report.vi"("window state (normal)"=T6."minimized", "display alerts? (F)"=FALSE, "report type"=Report_Type."Excel") -> ("report out"=w225:refnum<class "NI_report.lvclass">, "error out"=w227:errorcluster)  [unwired: 11 in]
                n90 = property on="Main Grading Table Disc 29" class="Tbl (strict)"() -> ("Value"=w228:string[][])  [unwired: 2 in, 2 out]
                n91 = call <vilib>:"Excel Easy Title.vi"("report in"=w225, "title"=w223, "start (0, 0)"=cluster{"row":i32, "column":i32} {"row"=0, "column"=2}, "font"=T4 {"font name"="Times New Roman", "font size"=24.0, "bold"=1, "italic"=0, "underline"=0, "strike through"=0, "font color"=16777216}, "error in (no error)"=w227) -> ("report out"=w224:refnum<class "NI_report.lvclass">, "error out"=w226:errorcluster)  [unwired: 8 in, 1 out]
                n92 = call-poly <vilib>:"Excel Easy Table.vi"("report in"=w224, "font"=T4 {"font name"="Times New Roman", "font size"=12.0, "bold"=0, "italic"=0, "underline"=0, "strike through"=0, "font color"=16777216}, "auto format (none)"=w212, "start (0, 0)"=cluster{"row":i32, "column":i32} {"row"=2, "column"=2}, "text data"=w228, "error in (no error)"=w226, "column headers"=string[] ["Date", "Time", "8-16mm", "10-14mm", "Disc Situation", "Control Mode", "Camera Situation", "Projector Situation"]) -> ("report out"=w208:refnum<class "NI_report.lvclass">, "error out"=w209:errorcluster)  [unwired: 4 in, 3 out]
                n93 = call-dynamic "Print Report.vi"("report in"=w208, "error in (no error)"=w209) -> ("report out"=w206:refnum<class "NI_report.lvclass">, "error out"=w207:errorcluster)  [unwired: 12 in]
                n94 = call-dynamic "Dispose Report.vi"("report in"=w206, "error in (no error)"=w207) -> ("error out"=w205:errorcluster)  [unwired: 13 in]
              }
              frame "Disc 05" {
                w236 = 1 items=["xlRangeAutoFormat3DEffects1"=13, "xlRangeAutoFormat3DEffects2"=14, "xlRangeAutoFormatAccounting1"=4, "xlRangeAutoFormatAccounting2"=5, "xlRangeAutoFormatAccounting3"=6, "xlRangeAutoFormatAccounting4"=17, "xlRangeAutoFormatClassic1"=1, "xlRangeAutoFormatClassic2"=2, "xlRangeAutoFormatClassic3"=3, "xlRangeAutoFormatColor1"=7, "xlRangeAutoFormatColor2"=8, "xlRangeAutoFormatColor3"=9, "xlRangeAutoFormatList1"=10, "xlRangeAutoFormatList2"=11, "xlRangeAutoFormatList3"=12, "xlRangeAutoFormatLocalFormat1"=15, "xlRangeAutoFormatLocalFormat2"=16, "xlRangeAutoFormatLocalFormat3"=19, "xlRangeAutoFormatLocalFormat4"=20, "xlRangeAutoFormatReport1"=21, "xlRangeAutoFormatReport2"=22, "xlRangeAutoFormatReport3"=23, "xlRangeAutoFormatReport4"=24, "xlRangeAutoFormatReport5"=25, "xlRangeAutoFormatReport6"=26, "xlRangeAutoFormatReport7"=27, "xlRangeAutoFormatReport8"=28, "xlRangeAutoFormatReport9"=29, "xlRangeAutoFormatReport10"=30, "xlRangeAutoFormatClassicPivotTable"=31, "xlRangeAutoFormatTable1"=32, "xlRangeAutoFormatTable2"=33, "xlRangeAutoFormatTable3"=34, "xlRangeAutoFormatTable4"=35, "xlRangeAutoFormatTable5"=36, "xlRangeAutoFormatTable6"=37, "xlRangeAutoFormatTable7"=38, "xlRangeAutoFormatTable8"=39, "xlRangeAutoFormatTable9"=40, "xlRangeAutoFormatTable10"=41, "xlRangeAutoFormatPTNone"=42, "xlRangeAutoFormatNone"=-4142, "xlRangeAutoFormatSimple"=-4154] ("auto format (none)")
                n95 = Get Date/Time In Seconds() -> (seconds since 1Jan1904=w245:timestamp)
                n96 = Format Date/Time String(time format string (%c)="%Y/%m/%d %H:%M:%S", seconds (now)=w245) -> (date/time string=w246:string)  [unwired: 1 in]
                n97 = Concatenate Strings("Grading Table Disc 30, Report Generated at " ("title"), w246) -> (w247:string)
                n98 = call <vilib>:"Create Report.vi"("window state (normal)"=T6."minimized", "display alerts? (F)"=FALSE, "report type"=Report_Type."Excel") -> ("report out"=w249:refnum<class "NI_report.lvclass">, "error out"=w251:errorcluster)  [unwired: 11 in]
                n99 = property on="Main Grading Table Disc 30" class="Tbl (strict)"() -> ("Value"=w252:string[][])  [unwired: 2 in, 2 out]
                n100 = call <vilib>:"Excel Easy Title.vi"("report in"=w249, "title"=w247, "start (0, 0)"=cluster{"row":i32, "column":i32} {"row"=0, "column"=0}, "font"=T4 {"font name"="Times New Roman", "font size"=24.0, "bold"=1, "italic"=0, "underline"=0, "strike through"=0, "font color"=16777216}, "error in (no error)"=w251) -> ("report out"=w248:refnum<class "NI_report.lvclass">, "error out"=w250:errorcluster)  [unwired: 8 in, 1 out]
                n101 = call-poly <vilib>:"Excel Easy Table.vi"("report in"=w248, "font"=T4 {"font name"="Times New Roman", "font size"=12.0, "bold"=0, "italic"=0, "underline"=0, "strike through"=0, "font color"=16777216}, "auto format (none)"=w236, "start (0, 0)"=cluster{"row":i32, "column":i32} {"row"=2, "column"=0}, "text data"=w252, "error in (no error)"=w250, "column headers"=string[] ["Date", "Time", "8-16mm", "10-14mm", "Disc Situation", "Control Mode", "Camera Situation", "Projector Situation"]) -> ("report out"=w232:refnum<class "NI_report.lvclass">, "error out"=w233:errorcluster)  [unwired: 4 in, 3 out]
                n102 = call-dynamic "Print Report.vi"("report in"=w232, "error in (no error)"=w233) -> ("report out"=w230:refnum<class "NI_report.lvclass">, "error out"=w231:errorcluster)  [unwired: 12 in]
                n103 = call-dynamic "Dispose Report.vi"("report in"=w230, "error in (no error)"=w231) -> ("error out"=w229:errorcluster)  [unwired: 13 in]
              }
            }
          }
          frame "Print 3" {
            w261 = 1 items=["xlRangeAutoFormat3DEffects1"=13, "xlRangeAutoFormat3DEffects2"=14, "xlRangeAutoFormatAccounting1"=4, "xlRangeAutoFormatAccounting2"=5, "xlRangeAutoFormatAccounting3"=6, "xlRangeAutoFormatAccounting4"=17, "xlRangeAutoFormatClassic1"=1, "xlRangeAutoFormatClassic2"=2, "xlRangeAutoFormatClassic3"=3, "xlRangeAutoFormatColor1"=7, "xlRangeAutoFormatColor2"=8, "xlRangeAutoFormatColor3"=9, "xlRangeAutoFormatList1"=10, "xlRangeAutoFormatList2"=11, "xlRangeAutoFormatList3"=12, "xlRangeAutoFormatLocalFormat1"=15, "xlRangeAutoFormatLocalFormat2"=16, "xlRangeAutoFormatLocalFormat3"=19, "xlRangeAutoFormatLocalFormat4"=20, "xlRangeAutoFormatReport1"=21, "xlRangeAutoFormatReport2"=22, "xlRangeAutoFormatReport3"=23, "xlRangeAutoFormatReport4"=24, "xlRangeAutoFormatReport5"=25, "xlRangeAutoFormatReport6"=26, "xlRangeAutoFormatReport7"=27, "xlRangeAutoFormatReport8"=28, "xlRangeAutoFormatReport9"=29, "xlRangeAutoFormatReport10"=30, "xlRangeAutoFormatClassicPivotTable"=31, "xlRangeAutoFormatTable1"=32, "xlRangeAutoFormatTable2"=33, "xlRangeAutoFormatTable3"=34, "xlRangeAutoFormatTable4"=35, "xlRangeAutoFormatTable5"=36, "xlRangeAutoFormatTable6"=37, "xlRangeAutoFormatTable7"=38, "xlRangeAutoFormatTable8"=39, "xlRangeAutoFormatTable9"=40, "xlRangeAutoFormatTable10"=41, "xlRangeAutoFormatPTNone"=42, "xlRangeAutoFormatNone"=-4142, "xlRangeAutoFormatSimple"=-4154] ("auto format (none)")
            n104 = call <vilib>:"Create Report.vi"("window state (normal)"=T6."minimized", "display alerts? (F)"=FALSE, "report type"=Report_Type."Excel") -> ("report out"=w269:refnum<class "NI_report.lvclass">, "error out"=w271:errorcluster)  [unwired: 11 in]
            n105 = call <vilib>:"Excel Easy Title.vi"("report in"=w269, "title"="Log Table", "start (0, 0)"=cluster{"row":i32, "column":i32} {"row"=0, "column"=0}, "font"=T4 {"font name"="Times New Roman", "font size"=24.0, "bold"=1, "italic"=0, "underline"=0, "strike through"=0, "font color"=16777216}, "error in (no error)"=w271) -> ("report out"=w268:refnum<class "NI_report.lvclass">, "error out"=w270:errorcluster)  [unwired: 8 in, 1 out]
            n106 = property on="Log Table" class="Tbl (strict)"() -> ("Value"=w272:string[][])  [unwired: 2 in, 2 out]
            n107 = call-poly <vilib>:"Excel Easy Table.vi"("report in"=w268, "font"=T4 {"font name"="Times New Roman", "font size"=12.0, "bold"=0, "italic"=0, "underline"=0, "strike through"=0, "font color"=16777216}, "auto format (none)"=w261, "start (0, 0)"=cluster{"row":i32, "column":i32} {"row"=2, "column"=0}, "text data"=w272, "error in (no error)"=w270, "column headers"=string[] ["Log Catalog", "Date", "Time", "Description"]) -> ("report out"=w257:refnum<class "NI_report.lvclass">, "error out"=w258:errorcluster)  [unwired: 4 in, 3 out]
            n108 = call-dynamic "Print Report.vi"("report in"=w257, "error in (no error)"=w258) -> ("report out"=w255:refnum<class "NI_report.lvclass">, "error out"=w256:errorcluster)  [unwired: 12 in]
            n109 = call-dynamic "Dispose Report.vi"("report in"=w255, "error in (no error)"=w256) -> ("error out"=w253:errorcluster)  [unwired: 13 in]
          }
        }
        n110 = shared-variable ".\\Maintenance.lvlib\\error_63"(w6) -> ()  [unwired: 1 in, 1 out]
      }
      event "Save 1", "Save 2", "Save 3": Mouse Down {
        n111 = event-data() -> ("CtlRef"=w275:refnum<vi>)  [unwired: 1 in, 7 out]
        n112 = property class="Bool (strict)"(reference=w275) -> ("Label.Text"=w274:string)  [unwired: 1 in, 2 out]
        n113 = case shown="\"Save 1\", Default" w274 {
          tunnel: [w276 w378 w480] -> w273
          frame "Save 1", Default {
            n114 = property on="Tab Control 2" class="TabCtl (strict)"() -> ("Value"=w277:T2)  [unwired: 2 in, 2 out]
            n115 = case shown="\"Disc 04\"" w277 {
              tunnel: [w278 w298 w318 w338 w358] -> w276
              frame "Disc 01", Default {
                w291 = 1 items=["xlRangeAutoFormat3DEffects1"=13, "xlRangeAutoFormat3DEffects2"=14, "xlRangeAutoFormatAccounting1"=4, "xlRangeAutoFormatAccounting2"=5, "xlRangeAutoFormatAccounting3"=6, "xlRangeAutoFormatAccounting4"=17, "xlRangeAutoFormatClassic1"=1, "xlRangeAutoFormatClassic2"=2, "xlRangeAutoFormatClassic3"=3, "xlRangeAutoFormatColor1"=7, "xlRangeAutoFormatColor2"=8, "xlRangeAutoFormatColor3"=9, "xlRangeAutoFormatList1"=10, "xlRangeAutoFormatList2"=11, "xlRangeAutoFormatList3"=12, "xlRangeAutoFormatLocalFormat1"=15, "xlRangeAutoFormatLocalFormat2"=16, "xlRangeAutoFormatLocalFormat3"=19, "xlRangeAutoFormatLocalFormat4"=20, "xlRangeAutoFormatReport1"=21, "xlRangeAutoFormatReport2"=22, "xlRangeAutoFormatReport3"=23, "xlRangeAutoFormatReport4"=24, "xlRangeAutoFormatReport5"=25, "xlRangeAutoFormatReport6"=26, "xlRangeAutoFormatReport7"=27, "xlRangeAutoFormatReport8"=28, "xlRangeAutoFormatReport9"=29, "xlRangeAutoFormatReport10"=30, "xlRangeAutoFormatClassicPivotTable"=31, "xlRangeAutoFormatTable1"=32, "xlRangeAutoFormatTable2"=33, "xlRangeAutoFormatTable3"=34, "xlRangeAutoFormatTable4"=35, "xlRangeAutoFormatTable5"=36, "xlRangeAutoFormatTable6"=37, "xlRangeAutoFormatTable7"=38, "xlRangeAutoFormatTable8"=39, "xlRangeAutoFormatTable9"=40, "xlRangeAutoFormatTable10"=41, "xlRangeAutoFormatPTNone"=42, "xlRangeAutoFormatNone"=-4142, "xlRangeAutoFormatSimple"=-4154] ("auto format (none)")
                n116 = Get Date/Time In Seconds() -> (seconds since 1Jan1904=w280:timestamp)
                n117 = Format Date/Time String(time format string (%c)="%Y/%m/%d %H:%M:%S", seconds (now)=w280) -> (date/time string=w281:string)  [unwired: 1 in]
                n118 = Concatenate Strings("Grading Table Disc 26, Report Generated at " ("title"), w281) -> (w282:string)
                n119 = call <vilib>:"Create Report.vi"("window state (normal)"=T6."maximized", "display alerts? (F)"=TRUE, "report type"=Report_Type."Excel") -> ("report out"=w287:refnum<class "NI_report.lvclass">, "error out"=w289:errorcluster)  [unwired: 11 in]
                n120 = property on="Grading Table Disc 26" class="Tbl (strict)"() -> ("Value"=w295:string[][])  [unwired: 2 in, 2 out]
                n121 = call <vilib>:"Excel Easy Title.vi"("report in"=w287, "title"=w282, "start (0, 0)"=cluster{"row":i32, "column":i32} {"row"=0, "column"=2}, "font"=T4 {"font name"="Times New Roman", "font size"=24.0, "bold"=1, "italic"=0, "underline"=0, "strike through"=0, "font color"=16777216}, "error in (no error)"=w289) -> ("report out"=w286:refnum<class "NI_report.lvclass">, "error out"=w288:errorcluster)  [unwired: 8 in, 1 out]
                n122 = call-poly <vilib>:"Excel Easy Table.vi"("report in"=w286, "font"=T4 {"font name"="Times New Roman", "font size"=12.0, "bold"=0, "italic"=0, "underline"=0, "strike through"=0, "font color"=16777216}, "auto format (none)"=w291, "start (0, 0)"=cluster{"row":i32, "column":i32} {"row"=2, "column"=2}, "text data"=w295, "error in (no error)"=w288, "column headers"=string[] ["Date", "Time", "<6.3mm", "6.3-8mm", "8-10mm", "10-12.5mm", "12.5-14mm", "14-16mm", "16-18mm", "18mm<", "Disc Situation", "Control Mode", "Camera Situation", "Projector Situation"]) -> ("error out"=w278:errorcluster)  [unwired: 4 in, 4 out]
              }
              frame "Disc 02" {
                w301 = 1 items=["xlRangeAutoFormat3DEffects1"=13, "xlRangeAutoFormat3DEffects2"=14, "xlRangeAutoFormatAccounting1"=4, "xlRangeAutoFormatAccounting2"=5, "xlRangeAutoFormatAccounting3"=6, "xlRangeAutoFormatAccounting4"=17, "xlRangeAutoFormatClassic1"=1, "xlRangeAutoFormatClassic2"=2, "xlRangeAutoFormatClassic3"=3, "xlRangeAutoFormatColor1"=7, "xlRangeAutoFormatColor2"=8, "xlRangeAutoFormatColor3"=9, "xlRangeAutoFormatList1"=10, "xlRangeAutoFormatList2"=11, "xlRangeAutoFormatList3"=12, "xlRangeAutoFormatLocalFormat1"=15, "xlRangeAutoFormatLocalFormat2"=16, "xlRangeAutoFormatLocalFormat3"=19, "xlRangeAutoFormatLocalFormat4"=20, "xlRangeAutoFormatReport1"=21, "xlRangeAutoFormatReport2"=22, "xlRangeAutoFormatReport3"=23, "xlRangeAutoFormatReport4"=24, "xlRangeAutoFormatReport5"=25, "xlRangeAutoFormatReport6"=26, "xlRangeAutoFormatReport7"=27, "xlRangeAutoFormatReport8"=28, "xlRangeAutoFormatReport9"=29, "xlRangeAutoFormatReport10"=30, "xlRangeAutoFormatClassicPivotTable"=31, "xlRangeAutoFormatTable1"=32, "xlRangeAutoFormatTable2"=33, "xlRangeAutoFormatTable3"=34, "xlRangeAutoFormatTable4"=35, "xlRangeAutoFormatTable5"=36, "xlRangeAutoFormatTable6"=37, "xlRangeAutoFormatTable7"=38, "xlRangeAutoFormatTable8"=39, "xlRangeAutoFormatTable9"=40, "xlRangeAutoFormatTable10"=41, "xlRangeAutoFormatPTNone"=42, "xlRangeAutoFormatNone"=-4142, "xlRangeAutoFormatSimple"=-4154] ("auto format (none)")
                n123 = Get Date/Time In Seconds() -> (seconds since 1Jan1904=w310:timestamp)
                n124 = Format Date/Time String(time format string (%c)="%Y/%m/%d %H:%M:%S", seconds (now)=w310) -> (date/time string=w311:string)  [unwired: 1 in]
                n125 = Concatenate Strings("Grading Table Disc 27, Report Generated at " ("title"), w311) -> (w312:string)
                n126 = call <vilib>:"Create Report.vi"("window state (normal)"=T6."maximized", "display alerts? (F)"=TRUE, "report type"=Report_Type."Excel") -> ("report out"=w314:refnum<class "NI_report.lvclass">, "error out"=w316:errorcluster)  [unwired: 11 in]
                n127 = property on="Grading Table Disc 27" class="Tbl (strict)"() -> ("Value"=w317:string[][])  [unwired: 2 in, 2 out]
                n128 = call <vilib>:"Excel Easy Title.vi"("report in"=w314, "title"=w312, "start (0, 0)"=cluster{"row":i32, "column":i32} {"row"=0, "column"=2}, "font"=T4 {"font name"="Times New Roman", "font size"=24.0, "bold"=1, "italic"=0, "underline"=0, "strike through"=0, "font color"=16777216}, "error in (no error)"=w316) -> ("report out"=w313:refnum<class "NI_report.lvclass">, "error out"=w315:errorcluster)  [unwired: 8 in, 1 out]
                n129 = call-poly <vilib>:"Excel Easy Table.vi"("report in"=w313, "font"=T4 {"font name"="Times New Roman", "font size"=12.0, "bold"=0, "italic"=0, "underline"=0, "strike through"=0, "font color"=16777216}, "auto format (none)"=w301, "start (0, 0)"=cluster{"row":i32, "column":i32} {"row"=2, "column"=2}, "text data"=w317, "error in (no error)"=w315, "column headers"=string[] ["Date", "Time", "<6.3mm", "6.3-8mm", "8-10mm", "10-12.5mm", "12.5-14mm", "14-16mm", "16-18mm", "18mm<", "Disc Situation", "Control Mode", "Camera Situation", "Projector Situation"]) -> ("error out"=w298:errorcluster)  [unwired: 4 in, 4 out]
              }
              frame "Disc 03" {
                w321 = 1 items=["xlRangeAutoFormat3DEffects1"=13, "xlRangeAutoFormat3DEffects2"=14, "xlRangeAutoFormatAccounting1"=4, "xlRangeAutoFormatAccounting2"=5, "xlRangeAutoFormatAccounting3"=6, "xlRangeAutoFormatAccounting4"=17, "xlRangeAutoFormatClassic1"=1, "xlRangeAutoFormatClassic2"=2, "xlRangeAutoFormatClassic3"=3, "xlRangeAutoFormatColor1"=7, "xlRangeAutoFormatColor2"=8, "xlRangeAutoFormatColor3"=9, "xlRangeAutoFormatList1"=10, "xlRangeAutoFormatList2"=11, "xlRangeAutoFormatList3"=12, "xlRangeAutoFormatLocalFormat1"=15, "xlRangeAutoFormatLocalFormat2"=16, "xlRangeAutoFormatLocalFormat3"=19, "xlRangeAutoFormatLocalFormat4"=20, "xlRangeAutoFormatReport1"=21, "xlRangeAutoFormatReport2"=22, "xlRangeAutoFormatReport3"=23, "xlRangeAutoFormatReport4"=24, "xlRangeAutoFormatReport5"=25, "xlRangeAutoFormatReport6"=26, "xlRangeAutoFormatReport7"=27, "xlRangeAutoFormatReport8"=28, "xlRangeAutoFormatReport9"=29, "xlRangeAutoFormatReport10"=30, "xlRangeAutoFormatClassicPivotTable"=31, "xlRangeAutoFormatTable1"=32, "xlRangeAutoFormatTable2"=33, "xlRangeAutoFormatTable3"=34, "xlRangeAutoFormatTable4"=35, "xlRangeAutoFormatTable5"=36, "xlRangeAutoFormatTable6"=37, "xlRangeAutoFormatTable7"=38, "xlRangeAutoFormatTable8"=39, "xlRangeAutoFormatTable9"=40, "xlRangeAutoFormatTable10"=41, "xlRangeAutoFormatPTNone"=42, "xlRangeAutoFormatNone"=-4142, "xlRangeAutoFormatSimple"=-4154] ("auto format (none)")
                n130 = Get Date/Time In Seconds() -> (seconds since 1Jan1904=w330:timestamp)
                n131 = Format Date/Time String(time format string (%c)="%Y/%m/%d %H:%M:%S", seconds (now)=w330) -> (date/time string=w331:string)  [unwired: 1 in]
                n132 = Concatenate Strings("Grading Table Disc 28, Report Generated at " ("title"), w331) -> (w332:string)
                n133 = call <vilib>:"Create Report.vi"("window state (normal)"=T6."maximized", "display alerts? (F)"=TRUE, "report type"=Report_Type."Excel") -> ("report out"=w334:refnum<class "NI_report.lvclass">, "error out"=w336:errorcluster)  [unwired: 11 in]
                n134 = property on="Grading Table Disc 28" class="Tbl (strict)"() -> ("Value"=w337:string[][])  [unwired: 2 in, 2 out]
                n135 = call <vilib>:"Excel Easy Title.vi"("report in"=w334, "title"=w332, "start (0, 0)"=cluster{"row":i32, "column":i32} {"row"=0, "column"=2}, "font"=T4 {"font name"="Times New Roman", "font size"=24.0, "bold"=1, "italic"=0, "underline"=0, "strike through"=0, "font color"=16777216}, "error in (no error)"=w336) -> ("report out"=w333:refnum<class "NI_report.lvclass">, "error out"=w335:errorcluster)  [unwired: 8 in, 1 out]
                n136 = call-poly <vilib>:"Excel Easy Table.vi"("report in"=w333, "font"=T4 {"font name"="Times New Roman", "font size"=12.0, "bold"=0, "italic"=0, "underline"=0, "strike through"=0, "font color"=16777216}, "auto format (none)"=w321, "start (0, 0)"=cluster{"row":i32, "column":i32} {"row"=2, "column"=2}, "text data"=w337, "error in (no error)"=w335, "column headers"=string[] ["Date", "Time", "<6.3mm", "6.3-8mm", "8-10mm", "10-12.5mm", "12.5-14mm", "14-16mm", "16-18mm", "18mm<", "Disc Situation", "Control Mode", "Camera Situation", "Projector Situation"]) -> ("error out"=w318:errorcluster)  [unwired: 4 in, 4 out]
              }
              frame "Disc 04" {
                w341 = 1 items=["xlRangeAutoFormat3DEffects1"=13, "xlRangeAutoFormat3DEffects2"=14, "xlRangeAutoFormatAccounting1"=4, "xlRangeAutoFormatAccounting2"=5, "xlRangeAutoFormatAccounting3"=6, "xlRangeAutoFormatAccounting4"=17, "xlRangeAutoFormatClassic1"=1, "xlRangeAutoFormatClassic2"=2, "xlRangeAutoFormatClassic3"=3, "xlRangeAutoFormatColor1"=7, "xlRangeAutoFormatColor2"=8, "xlRangeAutoFormatColor3"=9, "xlRangeAutoFormatList1"=10, "xlRangeAutoFormatList2"=11, "xlRangeAutoFormatList3"=12, "xlRangeAutoFormatLocalFormat1"=15, "xlRangeAutoFormatLocalFormat2"=16, "xlRangeAutoFormatLocalFormat3"=19, "xlRangeAutoFormatLocalFormat4"=20, "xlRangeAutoFormatReport1"=21, "xlRangeAutoFormatReport2"=22, "xlRangeAutoFormatReport3"=23, "xlRangeAutoFormatReport4"=24, "xlRangeAutoFormatReport5"=25, "xlRangeAutoFormatReport6"=26, "xlRangeAutoFormatReport7"=27, "xlRangeAutoFormatReport8"=28, "xlRangeAutoFormatReport9"=29, "xlRangeAutoFormatReport10"=30, "xlRangeAutoFormatClassicPivotTable"=31, "xlRangeAutoFormatTable1"=32, "xlRangeAutoFormatTable2"=33, "xlRangeAutoFormatTable3"=34, "xlRangeAutoFormatTable4"=35, "xlRangeAutoFormatTable5"=36, "xlRangeAutoFormatTable6"=37, "xlRangeAutoFormatTable7"=38, "xlRangeAutoFormatTable8"=39, "xlRangeAutoFormatTable9"=40, "xlRangeAutoFormatTable10"=41, "xlRangeAutoFormatPTNone"=42, "xlRangeAutoFormatNone"=-4142, "xlRangeAutoFormatSimple"=-4154] ("auto format (none)")
                n137 = Get Date/Time In Seconds() -> (seconds since 1Jan1904=w350:timestamp)
                n138 = Format Date/Time String(time format string (%c)="%Y/%m/%d %H:%M:%S", seconds (now)=w350) -> (date/time string=w351:string)  [unwired: 1 in]
                n139 = Concatenate Strings("Grading Table Disc 29, Report Generated at " ("title"), w351) -> (w352:string)
                n140 = call <vilib>:"Create Report.vi"("window state (normal)"=T6."maximized", "display alerts? (F)"=TRUE, "report type"=Report_Type."Excel") -> ("report out"=w354:refnum<class "NI_report.lvclass">, "error out"=w356:errorcluster)  [unwired: 11 in]
                n141 = property on="Grading Table Disc 29" class="Tbl (strict)"() -> ("Value"=w357:string[][])  [unwired: 2 in, 2 out]
                n142 = call <vilib>:"Excel Easy Title.vi"("report in"=w354, "title"=w352, "start (0, 0)"=cluster{"row":i32, "column":i32} {"row"=0, "column"=2}, "font"=T4 {"font name"="Times New Roman", "font size"=24.0, "bold"=1, "italic"=0, "underline"=0, "strike through"=0, "font color"=16777216}, "error in (no error)"=w356) -> ("report out"=w353:refnum<class "NI_report.lvclass">, "error out"=w355:errorcluster)  [unwired: 8 in, 1 out]
                n143 = call-poly <vilib>:"Excel Easy Table.vi"("report in"=w353, "font"=T4 {"font name"="Times New Roman", "font size"=12.0, "bold"=0, "italic"=0, "underline"=0, "strike through"=0, "font color"=16777216}, "auto format (none)"=w341, "start (0, 0)"=cluster{"row":i32, "column":i32} {"row"=2, "column"=2}, "text data"=w357, "error in (no error)"=w355, "column headers"=string[] ["Date", "Time", "<6.3mm", "6.3-8mm", "8-10mm", "10-12.5mm", "12.5-14mm", "14-16mm", "16-18mm", "18mm<", "Disc Situation", "Control Mode", "Camera Situation", "Projector Situation"]) -> ("error out"=w338:errorcluster)  [unwired: 4 in, 4 out]
              }
              frame "Disc 05" {
                w361 = 1 items=["xlRangeAutoFormat3DEffects1"=13, "xlRangeAutoFormat3DEffects2"=14, "xlRangeAutoFormatAccounting1"=4, "xlRangeAutoFormatAccounting2"=5, "xlRangeAutoFormatAccounting3"=6, "xlRangeAutoFormatAccounting4"=17, "xlRangeAutoFormatClassic1"=1, "xlRangeAutoFormatClassic2"=2, "xlRangeAutoFormatClassic3"=3, "xlRangeAutoFormatColor1"=7, "xlRangeAutoFormatColor2"=8, "xlRangeAutoFormatColor3"=9, "xlRangeAutoFormatList1"=10, "xlRangeAutoFormatList2"=11, "xlRangeAutoFormatList3"=12, "xlRangeAutoFormatLocalFormat1"=15, "xlRangeAutoFormatLocalFormat2"=16, "xlRangeAutoFormatLocalFormat3"=19, "xlRangeAutoFormatLocalFormat4"=20, "xlRangeAutoFormatReport1"=21, "xlRangeAutoFormatReport2"=22, "xlRangeAutoFormatReport3"=23, "xlRangeAutoFormatReport4"=24, "xlRangeAutoFormatReport5"=25, "xlRangeAutoFormatReport6"=26, "xlRangeAutoFormatReport7"=27, "xlRangeAutoFormatReport8"=28, "xlRangeAutoFormatReport9"=29, "xlRangeAutoFormatReport10"=30, "xlRangeAutoFormatClassicPivotTable"=31, "xlRangeAutoFormatTable1"=32, "xlRangeAutoFormatTable2"=33, "xlRangeAutoFormatTable3"=34, "xlRangeAutoFormatTable4"=35, "xlRangeAutoFormatTable5"=36, "xlRangeAutoFormatTable6"=37, "xlRangeAutoFormatTable7"=38, "xlRangeAutoFormatTable8"=39, "xlRangeAutoFormatTable9"=40, "xlRangeAutoFormatTable10"=41, "xlRangeAutoFormatPTNone"=42, "xlRangeAutoFormatNone"=-4142, "xlRangeAutoFormatSimple"=-4154] ("auto format (none)")
                n144 = Get Date/Time In Seconds() -> (seconds since 1Jan1904=w370:timestamp)
                n145 = Format Date/Time String(time format string (%c)="%Y/%m/%d %H:%M:%S", seconds (now)=w370) -> (date/time string=w371:string)  [unwired: 1 in]
                n146 = Concatenate Strings("Grading Table Disc 30, Report Generated at " ("title"), w371) -> (w372:string)
                n147 = call <vilib>:"Create Report.vi"("window state (normal)"=T6."maximized", "display alerts? (F)"=TRUE, "report type"=Report_Type."Excel") -> ("report out"=w374:refnum<class "NI_report.lvclass">, "error out"=w376:errorcluster)  [unwired: 11 in]
                n148 = property on="Grading Table Disc 30" class="Tbl (strict)"() -> ("Value"=w377:string[][])  [unwired: 2 in, 2 out]
                n149 = call <vilib>:"Excel Easy Title.vi"("report in"=w374, "title"=w372, "start (0, 0)"=cluster{"row":i32, "column":i32} {"row"=0, "column"=2}, "font"=T4 {"font name"="Times New Roman", "font size"=24.0, "bold"=1, "italic"=0, "underline"=0, "strike through"=0, "font color"=16777216}, "error in (no error)"=w376) -> ("report out"=w373:refnum<class "NI_report.lvclass">, "error out"=w375:errorcluster)  [unwired: 8 in, 1 out]
                n150 = call-poly <vilib>:"Excel Easy Table.vi"("report in"=w373, "font"=T4 {"font name"="Times New Roman", "font size"=12.0, "bold"=0, "italic"=0, "underline"=0, "strike through"=0, "font color"=16777216}, "auto format (none)"=w361, "start (0, 0)"=cluster{"row":i32, "column":i32} {"row"=2, "column"=2}, "text data"=w377, "error in (no error)"=w375, "column headers"=string[] ["Date", "Time", "<6.3mm", "6.3-8mm", "8-10mm", "10-12.5mm", "12.5-14mm", "14-16mm", "16-18mm", "18mm<", "Disc Situation", "Control Mode", "Camera Situation", "Projector Situation"]) -> ("error out"=w358:errorcluster)  [unwired: 4 in, 4 out]
              }
            }
          }
          frame "Save 2" {
            n151 = property on="Tab Control 3" class="TabCtl (strict)"() -> ("Value"=w379:T2)  [unwired: 2 in, 2 out]
            n152 = case shown="\"Disc 01\", Default" w379 {
              tunnel: [w380 w400 w420 w440 w460] -> w378
              frame "Disc 01", Default {
                w394 = 1 items=["xlRangeAutoFormat3DEffects1"=13, "xlRangeAutoFormat3DEffects2"=14, "xlRangeAutoFormatAccounting1"=4, "xlRangeAutoFormatAccounting2"=5, "xlRangeAutoFormatAccounting3"=6, "xlRangeAutoFormatAccounting4"=17, "xlRangeAutoFormatClassic1"=1, "xlRangeAutoFormatClassic2"=2, "xlRangeAutoFormatClassic3"=3, "xlRangeAutoFormatColor1"=7, "xlRangeAutoFormatColor2"=8, "xlRangeAutoFormatColor3"=9, "xlRangeAutoFormatList1"=10, "xlRangeAutoFormatList2"=11, "xlRangeAutoFormatList3"=12, "xlRangeAutoFormatLocalFormat1"=15, "xlRangeAutoFormatLocalFormat2"=16, "xlRangeAutoFormatLocalFormat3"=19, "xlRangeAutoFormatLocalFormat4"=20, "xlRangeAutoFormatReport1"=21, "xlRangeAutoFormatReport2"=22, "xlRangeAutoFormatReport3"=23, "xlRangeAutoFormatReport4"=24, "xlRangeAutoFormatReport5"=25, "xlRangeAutoFormatReport6"=26, "xlRangeAutoFormatReport7"=27, "xlRangeAutoFormatReport8"=28, "xlRangeAutoFormatReport9"=29, "xlRangeAutoFormatReport10"=30, "xlRangeAutoFormatClassicPivotTable"=31, "xlRangeAutoFormatTable1"=32, "xlRangeAutoFormatTable2"=33, "xlRangeAutoFormatTable3"=34, "xlRangeAutoFormatTable4"=35, "xlRangeAutoFormatTable5"=36, "xlRangeAutoFormatTable6"=37, "xlRangeAutoFormatTable7"=38, "xlRangeAutoFormatTable8"=39, "xlRangeAutoFormatTable9"=40, "xlRangeAutoFormatTable10"=41, "xlRangeAutoFormatPTNone"=42, "xlRangeAutoFormatNone"=-4142, "xlRangeAutoFormatSimple"=-4154] ("auto format (none)")
                n153 = Get Date/Time In Seconds() -> (seconds since 1Jan1904=w383:timestamp)
                n154 = Format Date/Time String(time format string (%c)="%Y/%m/%d %H:%M:%S", seconds (now)=w383) -> (date/time string=w384:string)  [unwired: 1 in]
                n155 = Concatenate Strings("Grading Table Disc 26, Report Generated at " ("title"), w384) -> (w385:string)
                n156 = call <vilib>:"Create Report.vi"("window state (normal)"=T6."maximized", "display alerts? (F)"=TRUE, "report type"=Report_Type."Excel") -> ("report out"=w390:refnum<class "NI_report.lvclass">, "error out"=w392:errorcluster)  [unwired: 11 in]
                n157 = property on="Main Grading Table Disc 26" class="Tbl (strict)"() -> ("Value"=w397:string[][])  [unwired: 2 in, 2 out]
                n158 = call <vilib>:"Excel Easy Title.vi"("report in"=w390, "title"=w385, "start (0, 0)"=cluster{"row":i32, "column":i32} {"row"=0, "column"=2}, "font"=T4 {"font name"="Times New Roman", "font size"=24.0, "bold"=1, "italic"=0, "underline"=0, "strike through"=0, "font color"=16777216}, "error in (no error)"=w392) -> ("report out"=w389:refnum<class "NI_report.lvclass">, "error out"=w391:errorcluster)  [unwired: 8 in, 1 out]
                n159 = call-poly <vilib>:"Excel Easy Table.vi"("report in"=w389, "font"=T4 {"font name"="Times New Roman", "font size"=12.0, "bold"=0, "italic"=0, "underline"=0, "strike through"=0, "font color"=16777216}, "auto format (none)"=w394, "start (0, 0)"=cluster{"row":i32, "column":i32} {"row"=2, "column"=2}, "text data"=w397, "error in (no error)"=w391, "column headers"=string[] ["Date", "Time", "8-16mm", "10-14mm", "Disc Situation", "Control Mode", "Camera Situation", "Projector Situation"]) -> ("error out"=w380:errorcluster)  [unwired: 4 in, 4 out]
              }
              frame "Disc 02" {
                w403 = 1 items=["xlRangeAutoFormat3DEffects1"=13, "xlRangeAutoFormat3DEffects2"=14, "xlRangeAutoFormatAccounting1"=4, "xlRangeAutoFormatAccounting2"=5, "xlRangeAutoFormatAccounting3"=6, "xlRangeAutoFormatAccounting4"=17, "xlRangeAutoFormatClassic1"=1, "xlRangeAutoFormatClassic2"=2, "xlRangeAutoFormatClassic3"=3, "xlRangeAutoFormatColor1"=7, "xlRangeAutoFormatColor2"=8, "xlRangeAutoFormatColor3"=9, "xlRangeAutoFormatList1"=10, "xlRangeAutoFormatList2"=11, "xlRangeAutoFormatList3"=12, "xlRangeAutoFormatLocalFormat1"=15, "xlRangeAutoFormatLocalFormat2"=16, "xlRangeAutoFormatLocalFormat3"=19, "xlRangeAutoFormatLocalFormat4"=20, "xlRangeAutoFormatReport1"=21, "xlRangeAutoFormatReport2"=22, "xlRangeAutoFormatReport3"=23, "xlRangeAutoFormatReport4"=24, "xlRangeAutoFormatReport5"=25, "xlRangeAutoFormatReport6"=26, "xlRangeAutoFormatReport7"=27, "xlRangeAutoFormatReport8"=28, "xlRangeAutoFormatReport9"=29, "xlRangeAutoFormatReport10"=30, "xlRangeAutoFormatClassicPivotTable"=31, "xlRangeAutoFormatTable1"=32, "xlRangeAutoFormatTable2"=33, "xlRangeAutoFormatTable3"=34, "xlRangeAutoFormatTable4"=35, "xlRangeAutoFormatTable5"=36, "xlRangeAutoFormatTable6"=37, "xlRangeAutoFormatTable7"=38, "xlRangeAutoFormatTable8"=39, "xlRangeAutoFormatTable9"=40, "xlRangeAutoFormatTable10"=41, "xlRangeAutoFormatPTNone"=42, "xlRangeAutoFormatNone"=-4142, "xlRangeAutoFormatSimple"=-4154] ("auto format (none)")
                n160 = Get Date/Time In Seconds() -> (seconds since 1Jan1904=w412:timestamp)
                n161 = Format Date/Time String(time format string (%c)="%Y/%m/%d %H:%M:%S", seconds (now)=w412) -> (date/time string=w413:string)  [unwired: 1 in]
                n162 = Concatenate Strings("Grading Table Disc 27, Report Generated at " ("title"), w413) -> (w414:string)
                n163 = call <vilib>:"Create Report.vi"("window state (normal)"=T6."maximized", "display alerts? (F)"=TRUE, "report type"=Report_Type."Excel") -> ("report out"=w416:refnum<class "NI_report.lvclass">, "error out"=w418:errorcluster)  [unwired: 11 in]
                n164 = property on="Main Grading Table Disc 27" class="Tbl (strict)"() -> ("Value"=w419:string[][])  [unwired: 2 in, 2 out]
                n165 = call <vilib>:"Excel Easy Title.vi"("report in"=w416, "title"=w414, "start (0, 0)"=cluster{"row":i32, "column":i32} {"row"=0, "column"=2}, "font"=T4 {"font name"="Times New Roman", "font size"=24.0, "bold"=1, "italic"=0, "underline"=0, "strike through"=0, "font color"=16777216}, "error in (no error)"=w418) -> ("report out"=w415:refnum<class "NI_report.lvclass">, "error out"=w417:errorcluster)  [unwired: 8 in, 1 out]
                n166 = call-poly <vilib>:"Excel Easy Table.vi"("report in"=w415, "font"=T4 {"font name"="Times New Roman", "font size"=12.0, "bold"=0, "italic"=0, "underline"=0, "strike through"=0, "font color"=16777216}, "auto format (none)"=w403, "start (0, 0)"=cluster{"row":i32, "column":i32} {"row"=2, "column"=2}, "text data"=w419, "error in (no error)"=w417, "column headers"=string[] ["Date", "Time", "8-16mm", "10-14mm", "Disc Situation", "Control Mode", "Camera Situation", "Projector Situation"]) -> ("error out"=w400:errorcluster)  [unwired: 4 in, 4 out]
              }
              frame "Disc 03" {
                w423 = 1 items=["xlRangeAutoFormat3DEffects1"=13, "xlRangeAutoFormat3DEffects2"=14, "xlRangeAutoFormatAccounting1"=4, "xlRangeAutoFormatAccounting2"=5, "xlRangeAutoFormatAccounting3"=6, "xlRangeAutoFormatAccounting4"=17, "xlRangeAutoFormatClassic1"=1, "xlRangeAutoFormatClassic2"=2, "xlRangeAutoFormatClassic3"=3, "xlRangeAutoFormatColor1"=7, "xlRangeAutoFormatColor2"=8, "xlRangeAutoFormatColor3"=9, "xlRangeAutoFormatList1"=10, "xlRangeAutoFormatList2"=11, "xlRangeAutoFormatList3"=12, "xlRangeAutoFormatLocalFormat1"=15, "xlRangeAutoFormatLocalFormat2"=16, "xlRangeAutoFormatLocalFormat3"=19, "xlRangeAutoFormatLocalFormat4"=20, "xlRangeAutoFormatReport1"=21, "xlRangeAutoFormatReport2"=22, "xlRangeAutoFormatReport3"=23, "xlRangeAutoFormatReport4"=24, "xlRangeAutoFormatReport5"=25, "xlRangeAutoFormatReport6"=26, "xlRangeAutoFormatReport7"=27, "xlRangeAutoFormatReport8"=28, "xlRangeAutoFormatReport9"=29, "xlRangeAutoFormatReport10"=30, "xlRangeAutoFormatClassicPivotTable"=31, "xlRangeAutoFormatTable1"=32, "xlRangeAutoFormatTable2"=33, "xlRangeAutoFormatTable3"=34, "xlRangeAutoFormatTable4"=35, "xlRangeAutoFormatTable5"=36, "xlRangeAutoFormatTable6"=37, "xlRangeAutoFormatTable7"=38, "xlRangeAutoFormatTable8"=39, "xlRangeAutoFormatTable9"=40, "xlRangeAutoFormatTable10"=41, "xlRangeAutoFormatPTNone"=42, "xlRangeAutoFormatNone"=-4142, "xlRangeAutoFormatSimple"=-4154] ("auto format (none)")
                n167 = Get Date/Time In Seconds() -> (seconds since 1Jan1904=w432:timestamp)
                n168 = Format Date/Time String(time format string (%c)="%Y/%m/%d %H:%M:%S", seconds (now)=w432) -> (date/time string=w433:string)  [unwired: 1 in]
                n169 = Concatenate Strings("Grading Table Disc 28, Report Generated at " ("title"), w433) -> (w434:string)
                n170 = call <vilib>:"Create Report.vi"("window state (normal)"=T6."maximized", "display alerts? (F)"=TRUE, "report type"=Report_Type."Excel") -> ("report out"=w436:refnum<class "NI_report.lvclass">, "error out"=w438:errorcluster)  [unwired: 11 in]
                n171 = property on="Main Grading Table Disc 28" class="Tbl (strict)"() -> ("Value"=w439:string[][])  [unwired: 2 in, 2 out]
                n172 = call <vilib>:"Excel Easy Title.vi"("report in"=w436, "title"=w434, "start (0, 0)"=cluster{"row":i32, "column":i32} {"row"=0, "column"=2}, "font"=T4 {"font name"="Times New Roman", "font size"=24.0, "bold"=1, "italic"=0, "underline"=0, "strike through"=0, "font color"=16777216}, "error in (no error)"=w438) -> ("report out"=w435:refnum<class "NI_report.lvclass">, "error out"=w437:errorcluster)  [unwired: 8 in, 1 out]
                n173 = call-poly <vilib>:"Excel Easy Table.vi"("report in"=w435, "font"=T4 {"font name"="Times New Roman", "font size"=12.0, "bold"=0, "italic"=0, "underline"=0, "strike through"=0, "font color"=16777216}, "auto format (none)"=w423, "start (0, 0)"=cluster{"row":i32, "column":i32} {"row"=2, "column"=2}, "text data"=w439, "error in (no error)"=w437, "column headers"=string[] ["Date", "Time", "8-16mm", "10-14mm", "Disc Situation", "Control Mode", "Camera Situation", "Projector Situation"]) -> ("error out"=w420:errorcluster)  [unwired: 4 in, 4 out]
              }
              frame "Disc 04" {
                w443 = 1 items=["xlRangeAutoFormat3DEffects1"=13, "xlRangeAutoFormat3DEffects2"=14, "xlRangeAutoFormatAccounting1"=4, "xlRangeAutoFormatAccounting2"=5, "xlRangeAutoFormatAccounting3"=6, "xlRangeAutoFormatAccounting4"=17, "xlRangeAutoFormatClassic1"=1, "xlRangeAutoFormatClassic2"=2, "xlRangeAutoFormatClassic3"=3, "xlRangeAutoFormatColor1"=7, "xlRangeAutoFormatColor2"=8, "xlRangeAutoFormatColor3"=9, "xlRangeAutoFormatList1"=10, "xlRangeAutoFormatList2"=11, "xlRangeAutoFormatList3"=12, "xlRangeAutoFormatLocalFormat1"=15, "xlRangeAutoFormatLocalFormat2"=16, "xlRangeAutoFormatLocalFormat3"=19, "xlRangeAutoFormatLocalFormat4"=20, "xlRangeAutoFormatReport1"=21, "xlRangeAutoFormatReport2"=22, "xlRangeAutoFormatReport3"=23, "xlRangeAutoFormatReport4"=24, "xlRangeAutoFormatReport5"=25, "xlRangeAutoFormatReport6"=26, "xlRangeAutoFormatReport7"=27, "xlRangeAutoFormatReport8"=28, "xlRangeAutoFormatReport9"=29, "xlRangeAutoFormatReport10"=30, "xlRangeAutoFormatClassicPivotTable"=31, "xlRangeAutoFormatTable1"=32, "xlRangeAutoFormatTable2"=33, "xlRangeAutoFormatTable3"=34, "xlRangeAutoFormatTable4"=35, "xlRangeAutoFormatTable5"=36, "xlRangeAutoFormatTable6"=37, "xlRangeAutoFormatTable7"=38, "xlRangeAutoFormatTable8"=39, "xlRangeAutoFormatTable9"=40, "xlRangeAutoFormatTable10"=41, "xlRangeAutoFormatPTNone"=42, "xlRangeAutoFormatNone"=-4142, "xlRangeAutoFormatSimple"=-4154] ("auto format (none)")
                n174 = Get Date/Time In Seconds() -> (seconds since 1Jan1904=w452:timestamp)
                n175 = Format Date/Time String(time format string (%c)="%Y/%m/%d %H:%M:%S", seconds (now)=w452) -> (date/time string=w453:string)  [unwired: 1 in]
                n176 = Concatenate Strings("Grading Table Disc 29, Report Generated at " ("title"), w453) -> (w454:string)
                n177 = call <vilib>:"Create Report.vi"("window state (normal)"=T6."maximized", "display alerts? (F)"=TRUE, "report type"=Report_Type."Excel") -> ("report out"=w456:refnum<class "NI_report.lvclass">, "error out"=w458:errorcluster)  [unwired: 11 in]
                n178 = property on="Main Grading Table Disc 29" class="Tbl (strict)"() -> ("Value"=w459:string[][])  [unwired: 2 in, 2 out]
                n179 = call <vilib>:"Excel Easy Title.vi"("report in"=w456, "title"=w454, "start (0, 0)"=cluster{"row":i32, "column":i32} {"row"=0, "column"=2}, "font"=T4 {"font name"="Times New Roman", "font size"=24.0, "bold"=1, "italic"=0, "underline"=0, "strike through"=0, "font color"=16777216}, "error in (no error)"=w458) -> ("report out"=w455:refnum<class "NI_report.lvclass">, "error out"=w457:errorcluster)  [unwired: 8 in, 1 out]
                n180 = call-poly <vilib>:"Excel Easy Table.vi"("report in"=w455, "font"=T4 {"font name"="Times New Roman", "font size"=12.0, "bold"=0, "italic"=0, "underline"=0, "strike through"=0, "font color"=16777216}, "auto format (none)"=w443, "start (0, 0)"=cluster{"row":i32, "column":i32} {"row"=2, "column"=2}, "text data"=w459, "error in (no error)"=w457, "column headers"=string[] ["Date", "Time", "8-16mm", "10-14mm", "Disc Situation", "Control Mode", "Camera Situation", "Projector Situation"]) -> ("error out"=w440:errorcluster)  [unwired: 4 in, 4 out]
              }
              frame "Disc 05" {
                w463 = 1 items=["xlRangeAutoFormat3DEffects1"=13, "xlRangeAutoFormat3DEffects2"=14, "xlRangeAutoFormatAccounting1"=4, "xlRangeAutoFormatAccounting2"=5, "xlRangeAutoFormatAccounting3"=6, "xlRangeAutoFormatAccounting4"=17, "xlRangeAutoFormatClassic1"=1, "xlRangeAutoFormatClassic2"=2, "xlRangeAutoFormatClassic3"=3, "xlRangeAutoFormatColor1"=7, "xlRangeAutoFormatColor2"=8, "xlRangeAutoFormatColor3"=9, "xlRangeAutoFormatList1"=10, "xlRangeAutoFormatList2"=11, "xlRangeAutoFormatList3"=12, "xlRangeAutoFormatLocalFormat1"=15, "xlRangeAutoFormatLocalFormat2"=16, "xlRangeAutoFormatLocalFormat3"=19, "xlRangeAutoFormatLocalFormat4"=20, "xlRangeAutoFormatReport1"=21, "xlRangeAutoFormatReport2"=22, "xlRangeAutoFormatReport3"=23, "xlRangeAutoFormatReport4"=24, "xlRangeAutoFormatReport5"=25, "xlRangeAutoFormatReport6"=26, "xlRangeAutoFormatReport7"=27, "xlRangeAutoFormatReport8"=28, "xlRangeAutoFormatReport9"=29, "xlRangeAutoFormatReport10"=30, "xlRangeAutoFormatClassicPivotTable"=31, "xlRangeAutoFormatTable1"=32, "xlRangeAutoFormatTable2"=33, "xlRangeAutoFormatTable3"=34, "xlRangeAutoFormatTable4"=35, "xlRangeAutoFormatTable5"=36, "xlRangeAutoFormatTable6"=37, "xlRangeAutoFormatTable7"=38, "xlRangeAutoFormatTable8"=39, "xlRangeAutoFormatTable9"=40, "xlRangeAutoFormatTable10"=41, "xlRangeAutoFormatPTNone"=42, "xlRangeAutoFormatNone"=-4142, "xlRangeAutoFormatSimple"=-4154] ("auto format (none)")
                n181 = Get Date/Time In Seconds() -> (seconds since 1Jan1904=w472:timestamp)
                n182 = Format Date/Time String(time format string (%c)="%Y/%m/%d %H:%M:%S", seconds (now)=w472) -> (date/time string=w473:string)  [unwired: 1 in]
                n183 = Concatenate Strings("Grading Table Disc 30, Report Generated at " ("title"), w473) -> (w474:string)
                n184 = call <vilib>:"Create Report.vi"("window state (normal)"=T6."maximized", "display alerts? (F)"=TRUE, "report type"=Report_Type."Excel") -> ("report out"=w476:refnum<class "NI_report.lvclass">, "error out"=w478:errorcluster)  [unwired: 11 in]
                n185 = property on="Main Grading Table Disc 30" class="Tbl (strict)"() -> ("Value"=w479:string[][])  [unwired: 2 in, 2 out]
                n186 = call <vilib>:"Excel Easy Title.vi"("report in"=w476, "title"=w474, "start (0, 0)"=cluster{"row":i32, "column":i32} {"row"=0, "column"=2}, "font"=T4 {"font name"="Times New Roman", "font size"=24.0, "bold"=1, "italic"=0, "underline"=0, "strike through"=0, "font color"=16777216}, "error in (no error)"=w478) -> ("report out"=w475:refnum<class "NI_report.lvclass">, "error out"=w477:errorcluster)  [unwired: 8 in, 1 out]
                n187 = call-poly <vilib>:"Excel Easy Table.vi"("report in"=w475, "font"=T4 {"font name"="Times New Roman", "font size"=12.0, "bold"=0, "italic"=0, "underline"=0, "strike through"=0, "font color"=16777216}, "auto format (none)"=w463, "start (0, 0)"=cluster{"row":i32, "column":i32} {"row"=2, "column"=2}, "text data"=w479, "error in (no error)"=w477, "column headers"=string[] ["Date", "Time", "8-16mm", "10-14mm", "Disc Situation", "Control Mode", "Camera Situation", "Projector Situation"]) -> ("error out"=w460:errorcluster)  [unwired: 4 in, 4 out]
              }
            }
          }
          frame "Save 3" {
            w483 = 1 items=["xlRangeAutoFormat3DEffects1"=13, "xlRangeAutoFormat3DEffects2"=14, "xlRangeAutoFormatAccounting1"=4, "xlRangeAutoFormatAccounting2"=5, "xlRangeAutoFormatAccounting3"=6, "xlRangeAutoFormatAccounting4"=17, "xlRangeAutoFormatClassic1"=1, "xlRangeAutoFormatClassic2"=2, "xlRangeAutoFormatClassic3"=3, "xlRangeAutoFormatColor1"=7, "xlRangeAutoFormatColor2"=8, "xlRangeAutoFormatColor3"=9, "xlRangeAutoFormatList1"=10, "xlRangeAutoFormatList2"=11, "xlRangeAutoFormatList3"=12, "xlRangeAutoFormatLocalFormat1"=15, "xlRangeAutoFormatLocalFormat2"=16, "xlRangeAutoFormatLocalFormat3"=19, "xlRangeAutoFormatLocalFormat4"=20, "xlRangeAutoFormatReport1"=21, "xlRangeAutoFormatReport2"=22, "xlRangeAutoFormatReport3"=23, "xlRangeAutoFormatReport4"=24, "xlRangeAutoFormatReport5"=25, "xlRangeAutoFormatReport6"=26, "xlRangeAutoFormatReport7"=27, "xlRangeAutoFormatReport8"=28, "xlRangeAutoFormatReport9"=29, "xlRangeAutoFormatReport10"=30, "xlRangeAutoFormatClassicPivotTable"=31, "xlRangeAutoFormatTable1"=32, "xlRangeAutoFormatTable2"=33, "xlRangeAutoFormatTable3"=34, "xlRangeAutoFormatTable4"=35, "xlRangeAutoFormatTable5"=36, "xlRangeAutoFormatTable6"=37, "xlRangeAutoFormatTable7"=38, "xlRangeAutoFormatTable8"=39, "xlRangeAutoFormatTable9"=40, "xlRangeAutoFormatTable10"=41, "xlRangeAutoFormatPTNone"=42, "xlRangeAutoFormatNone"=-4142, "xlRangeAutoFormatSimple"=-4154] ("auto format (none)")
            n188 = Get Date/Time In Seconds() -> (seconds since 1Jan1904=w492:timestamp)
            n189 = Format Date/Time String(time format string (%c)="%Y/%m/%d %H:%M:%S", seconds (now)=w492) -> (date/time string=w493:string)  [unwired: 1 in]
            n190 = Concatenate Strings("Log Table, Report Generated at " ("title"), w493) -> (w494:string)
            n191 = call <vilib>:"Create Report.vi"("window state (normal)"=T6."maximized", "display alerts? (F)"=TRUE, "report type"=Report_Type."Excel") -> ("report out"=w496:refnum<class "NI_report.lvclass">, "error out"=w498:errorcluster)  [unwired: 11 in]
            n192 = call <vilib>:"Excel Easy Title.vi"("report in"=w496, "title"=w494, "start (0, 0)"=cluster{"row":i32, "column":i32} {"row"=0, "column"=2}, "font"=T4 {"font name"="Times New Roman", "font size"=24.0, "bold"=1, "italic"=0, "underline"=0, "strike through"=0, "font color"=16777216}, "error in (no error)"=w498) -> ("report out"=w495:refnum<class "NI_report.lvclass">, "error out"=w497:errorcluster)  [unwired: 8 in, 1 out]
            n193 = property on="Log Table" class="Tbl (strict)"() -> ("Value"=w499:string[][])  [unwired: 2 in, 2 out]
            n194 = call-poly <vilib>:"Excel Easy Table.vi"("report in"=w495, "font"=T4 {"font name"="Times New Roman", "font size"=12.0, "bold"=0, "italic"=0, "underline"=0, "strike through"=0, "font color"=16777216}, "auto format (none)"=w483, "start (0, 0)"=cluster{"row":i32, "column":i32} {"row"=2, "column"=2}, "text data"=w499, "error in (no error)"=w497, "column headers"=string[] ["Log Catalog", "Date", "Time", "Description"]) -> ("error out"=w480:errorcluster)  [unwired: 4 in, 4 out]
          }
        }
        n195 = shared-variable ".\\Maintenance.lvlib\\error_64"(w273) -> ()  [unwired: 1 in, 1 out]
      }
      event "Search 1", "Search 2": Mouse Down {
        n196 = event-data() -> ()  [unwired: 1 in, 8 out]
        n197 = flat-sequence {
          tunnel: [w503] -> w500
          tunnel: w500 -> [w524]
          frame #0 {
            n198 = call "grading table searching.vi"() -> ()  [unwired: 12 in]
          }
          frame #1 {
            n199 = case shown="\"Grading Table\", Default" "Tab Control 1" {
              tunnel: [w508 w516] -> w504
              frame "Grading Table", Default {
                n200 = case shown="\"Disc 06\"" "Tab Control 2" {
                  tunnel: ["grading_disc_01" ("Connection Name") "grading_disc_02" ("Connection Name") "grading_disc_03" ("Connection Name") "grading_disc_04" ("Connection Name") "grading_disc_05" ("Connection Name") "grading_disc_06" ("Connection Name")] -> w508
                  frame "Disc 01", Default {
                  }
                  frame "Disc 02" {
                  }
                  frame "Disc 03" {
                  }
                  frame "Disc 04" {
                  }
                  frame "Disc 05" {
                  }
                  frame "Disc 06" {
                  }
                }
              }
              frame "Main Grading Table" {
                n201 = case shown="\"Disc 06\"" "Tab Control 3" {
                  tunnel: ["main_grading_group_disc_01" ("Connection Name") "main_grading_group_disc_02" ("Connection Name") "main_grading_group_disc_03" ("Connection Name") "main_grading_group_disc_04" ("Connection Name") "main_grading_group_disc_05" ("Connection Name") "main_grading_group_disc_06" ("Connection Name")] -> w516
                  frame "Disc 01", Default {
                  }
                  frame "Disc 02" {
                  }
                  frame "Disc 03" {
                  }
                  frame "Disc 04" {
                  }
                  frame "Disc 05" {
                  }
                  frame "Disc 06" {
                  }
                }
              }
            }
            n202 = shared-variable ".\\database.lvlib\\Query String"() -> (w507:string, error out=w502:errorcluster)  [unwired: 1 in]
            n203 = call "Query.vi"("Condition"=w507, "Error in"=w502, "Table Name"=w504, "Connection Name"="dsgs") -> ("Error out"=w501:errorcluster, "data"=w503:string[][])
            n204 = shared-variable ".\\Maintenance.lvlib\\error_65"(w501) -> ()  [unwired: 1 in, 1 out]
          }
          frame #2 {
            n205 = property on="Tab Control 1" class="TabCtl (strict)"() -> ("Value"=w525:T1)  [unwired: 2 in, 2 out]
            n206 = case shown="\"Main Grading Table\"" w525 {
              tunnel: w524 -> [w526 w546]
              frame "Grading Table", Default {
                n207 = property on="Tab Control 2" class="TabCtl (strict)"() -> ("Value"=w527:T2)  [unwired: 2 in, 2 out]
                n208 = case shown="\"Disc 06\"" w527 {
                  tunnel: w526 -> [w530 w532 w535 w538 w541 w544]
                  frame "Disc 01", Default {
                    n209 = Array Subset(array=w530, index (col)=1 ("index")) -> (→"Grading Table Disc 26":string[][])  [unwired: 3 in]
                  }
                  frame "Disc 02" {
                    n210 = Array Subset(array=w532, index (col)=1 ("index")) -> (→"Grading Table Disc 27":string[][])  [unwired: 3 in]
                  }
                  frame "Disc 03" {
                    n211 = Array Subset(array=w535, index (col)=1 ("index")) -> (→"Grading Table Disc 28":string[][])  [unwired: 3 in]
                  }
                  frame "Disc 04" {
                    n212 = Array Subset(array=w538, index (col)=1 ("index")) -> (→"Grading Table Disc 29":string[][])  [unwired: 3 in]
                  }
                  frame "Disc 05" {
                    n213 = Array Subset(array=w541, index (col)=1 ("index")) -> (→"Grading Table Disc 30":string[][])  [unwired: 3 in]
                  }
                  frame "Disc 06" {
                    n214 = Array Subset(array=w544, index (col)=1 ("index")) -> (→"Grading Table Disc 06":string[][])  [unwired: 3 in]
                  }
                }
              }
              frame "Main Grading Table" {
                n215 = property on="Tab Control 3" class="TabCtl (strict)"() -> ("Value"=w547:T2)  [unwired: 2 in, 2 out]
                n216 = case shown="\"Disc 06\"" w547 {
                  tunnel: w546 -> [w549 w552 w555 w558 w561 w564]
                  frame "Disc 01", Default {
                    n217 = Array Subset(array=w549, index (col)=1 ("index")) -> (→"Main Grading Table Disc 26":string[][])  [unwired: 3 in]
                  }
                  frame "Disc 02" {
                    n218 = Array Subset(array=w552, index (col)=1 ("index")) -> (→"Main Grading Table Disc 27":string[][])  [unwired: 3 in]
                  }
                  frame "Disc 03" {
                    n219 = Array Subset(array=w555, index (col)=1 ("index")) -> (→"Main Grading Table Disc 28":string[][])  [unwired: 3 in]
                  }
                  frame "Disc 04" {
                    n220 = Array Subset(array=w558, index (col)=1 ("index")) -> (→"Main Grading Table Disc 29":string[][])  [unwired: 3 in]
                  }
                  frame "Disc 05" {
                    n221 = Array Subset(array=w561, index (col)=1 ("index")) -> (→"Main Grading Table Disc 30":string[][])  [unwired: 3 in]
                  }
                  frame "Disc 06" {
                    n222 = Array Subset(array=w564, index (col)=1 ("index")) -> (→"Main Grading Table Disc 06":string[][])  [unwired: 3 in]
                  }
                }
              }
            }
          }
        }
      }
      event "Grading Table Disc 26", "Grading Table Disc 27", "Grading Table Disc 28", "Grading Table Disc 29", "Grading Table Disc 30": Mouse Down {
        n223 = event-data() -> ("CtlRef"=w573:refnum<vi>)  [unwired: 1 in, 7 out]
        n224 = property on="Property Node" class="Tbl (strict)"(reference=w573) -> ("Value"=w572:string[][], "Selection Start"=w575:T7)  [unwired: 1 in, 2 out]
        n225 = Unbundle By Name(w575) -> ("Row"=w570:i32)
        n226 = Matrix Size(0:w572) -> (1:w571:i32)  [unwired: 1 out]
        n227 = Greater Or Equal?(x=w571, y=w570) -> (x >= y?=w569:bool)
        n228 = Select(t=T7 {"Row"=1, "Column"=14} ("Selection Size"), s=w569, f=T7 {"Row"=0, "Column"=0}) -> (s? t:f=w567:T7)
        n229 = Bundle("Row"=w570, "Row"=0) -> (w577:cluster{"Row":i32, "Row":i32})  [unwired: 1 in]
        n230 = property on="Property Node" class="Tbl (strict)"(reference=w573, "Selection Color"=u32 16711680, "Selection Size"=w567, "Selection Start"=w577) -> ()  [unwired: 1 in, 2 out]
      }
      event "Main Grading Table Disc 26", "Main Grading Table Disc 27", "Main Grading Table Disc 28", "Main Grading Table Disc 29", "Main Grading Table Disc 30": Mouse Down {
        n231 = event-data() -> ("CtlRef"=w585:refnum<vi>)  [unwired: 1 in, 7 out]
        n232 = property on="Property Node" class="Tbl (strict)"(reference=w585) -> ("Value"=w580:string[][], "Selection Start"=w587:T7)  [unwired: 1 in, 2 out]
        n233 = Unbundle By Name(w587) -> ("Row"=w578:i32)
        n234 = Matrix Size(0:w580) -> (1:w584:i32)  [unwired: 1 out]
        n235 = Greater Or Equal?(x=w584, y=w578) -> (x >= y?=w583:bool)
        n236 = Bundle("Row"=w578, "Row"=0) -> (w589:cluster{"Row":i32, "Row":i32})  [unwired: 1 in]
        n237 = Select(t=T7 {"Row"=1, "Column"=8} ("Selection Size"), s=w583, f=T7 {"Row"=0, "Column"=0}) -> (s? t:f=w579:T7)
        n238 = property on="Property Node" class="Tbl (strict)"(reference=w585, "Selection Color"=u32 16711680, "Selection Size"=w579, "Selection Start"=w589) -> ()  [unwired: 1 in, 2 out]
      }
      event "Log Catalog Table", "Log Table", "User Table": Mouse Down {
        n239 = event-data() -> ("CtlRef"=w597:refnum<vi>)  [unwired: 1 in, 7 out]
        n240 = property on="Property Node" class="Tbl (strict)"(reference=w597) -> ("Value"=w592:string[][], "Selection Start"=w599:T7)  [unwired: 1 in, 2 out]
        n241 = Unbundle By Name(w599) -> ("Row"=w591:i32)
        n242 = Matrix Size(0:w592) -> (1:w596:i32)  [unwired: 1 out]
        n243 = Greater Or Equal?(x=w596, y=w591) -> (x >= y?=w595:bool)
        n244 = Bundle("Row"=w591, "Row"=0) -> (w601:cluster{"Row":i32, "Row":i32})  [unwired: 1 in]
        n245 = Select(t=T7 {"Row"=1, "Column"=4} ("Selection Size"), s=w595, f=T7 {"Row"=0, "Column"=0}) -> (s? t:f=w590:T7)
        n246 = property on="Property Node" class="Tbl (strict)"(reference=w597, "Selection Color"=u32 16711680, "Selection Size"=w590, "Selection Start"=w601) -> ()  [unwired: 1 in, 2 out]
      }
      event "Search 3": Mouse Down {
        n247 = event-data() -> ()  [unwired: 1 in, 8 out]
        n248 = flat-sequence {
          frame #0 {
            n249 = call "log table searching.vi"() -> ()  [unwired: 12 in]
          }
          frame #1 {
            n250 = shared-variable ".\\database.lvlib\\Query String"() -> (w608:string, error out=w603:errorcluster)  [unwired: 1 in]
            n251 = call "Query.vi"("Condition"=w608, "Error in"=w603, "Table Name"="log_table", "Connection Name"="dsgs") -> ("Error out"=w602:errorcluster, "data"=w606:string[][])
            n252 = shared-variable ".\\Maintenance.lvlib\\error_66"(w602) -> ()  [unwired: 1 in, 1 out]
            n253 = Array Subset(array=w606, index (col)=1 ("index")) -> (→"Log Table":string[][])  [unwired: 3 in]
          }
        }
      }
      event "Tab Control 1": Mouse Down {
        n254 = event-data() -> ("CtlRef"=w611:refnum<vi>)  [unwired: 1 in, 7 out]
        n255 = property class="TabCtl (strict)"(reference=w611) -> ("Value"=w610:T1)  [unwired: 1 in, 2 out]
        n256 = case shown="\"User Table\", Default" w610 {
          frame "Log Table" {
            n257 = call "Query.vi"("Table Name"="log_catalog", "Connection Name"="dsgs") -> ("Error out"=w612:errorcluster, "data"=→"Log Catalog Table":string[][])  [unwired: 2 in]
            n258 = shared-variable ".\\Maintenance.lvlib\\error_67"(w612) -> ()  [unwired: 1 in, 1 out]
          }
          frame "User Table", Default {
            n259 = call "Query.vi"("Table Name"="user_table", "Connection Name"="dsgs") -> ("Error out"=w616:errorcluster, "data"=w624:string[][])  [unwired: 2 in]
            n260 = Index Array(array=w624, index (col) #1=0 ("disabled index (col)"), index (col) #3=3 ("index (col)")) -> (element #1=w621:string[], element #2=w620:string[], element #3=w619:string[])  [unwired: 4 in]
            n261 = shared-variable ".\\Maintenance.lvlib\\error_68"(w616) -> ()  [unwired: 1 in, 1 out]
            n262 = Build Array(w621, w620, w619) -> (w618:string[][])
            n263 = Transpose 2D Array(2D array=w618) -> (transposed array=→"User Table":string[][])
          }
        }
      }
      event Timeout {
        n264 = event-data() -> ()  [unwired: 1 in, 3 out]
        n265 = control-ref of="This VI"() -> (w627:refnum<vi>)
        n266 = shared-variable ".\\database.lvlib\\ReportThisVI"(w627) -> ()  [unwired: 1 in, 1 out]
      }
    }
  }
  n267 = property on="User Table" class="Tbl (strict)"("BuiltInMouseWheelSupport"=w1) -> ()  [unwired: 2 in, 2 out]
  n268 = property on="Log Table" class="Tbl (strict)"("BuiltInMouseWheelSupport"=w1) -> ()  [unwired: 2 in, 2 out]
  n269 = property on="Log Catalog Table" class="Tbl (strict)"("BuiltInMouseWheelSupport"=w1) -> ()  [unwired: 2 in, 2 out]
  n270 = property on="Grading Table Disc 26" class="Tbl (strict)"("BuiltInMouseWheelSupport"=w1) -> ()  [unwired: 2 in, 2 out]
  n271 = property on="Grading Table Disc 27" class="Tbl (strict)"("BuiltInMouseWheelSupport"=w1) -> ()  [unwired: 2 in, 2 out]
  n272 = property on="Grading Table Disc 28" class="Tbl (strict)"("BuiltInMouseWheelSupport"=w1) -> ()  [unwired: 2 in, 2 out]
  n273 = property on="Grading Table Disc 29" class="Tbl (strict)"("BuiltInMouseWheelSupport"=w1) -> ()  [unwired: 2 in, 2 out]
  n274 = property on="Grading Table Disc 30" class="Tbl (strict)"("BuiltInMouseWheelSupport"=w1) -> ()  [unwired: 2 in, 2 out]
  n275 = property on="Main Grading Table Disc 26" class="Tbl (strict)"("BuiltInMouseWheelSupport"=w1) -> ()  [unwired: 2 in, 2 out]
  n276 = property on="Main Grading Table Disc 27" class="Tbl (strict)"("BuiltInMouseWheelSupport"=w1) -> ()  [unwired: 2 in, 2 out]
  n277 = property on="Main Grading Table Disc 28" class="Tbl (strict)"("BuiltInMouseWheelSupport"=w1) -> ()  [unwired: 2 in, 2 out]
  n278 = property on="Main Grading Table Disc 29" class="Tbl (strict)"("BuiltInMouseWheelSupport"=w1) -> ()  [unwired: 2 in, 2 out]
  n279 = property on="Main Grading Table Disc 30" class="Tbl (strict)"("BuiltInMouseWheelSupport"=w1) -> ()  [unwired: 2 in, 2 out]
